vi "GetAction.vi"(0 "Check Condition":T16, 5 "Query Array":T17[](array[typedef]), 7 "input cluster":T1, 11 "error in (no error)":errorcluster) -> (3 "Compound AND":bool, 4 "Results Array":bool[](array[boolean]), 6 "Status Array Out":string[](array[string]), 13 "Convectron ATM Result Array":i32[](array[numeric]), 14 "Generate Event?":bool, 15 "error out":errorcluster)   [LabVIEW 2011]
uses:
  action_typdef.ctl
  Error codes.ctl
  MainCluster_typdef.ctl
  EC Status Named_typdef.ctl
  EC Statusboolarray2_typdef.ctl
  EC Statusboolarray3_typdef.ctl
  EC Statusboolarray1_typdef.ctl
  EC statusintegerarray_typdef.ctl
  EC statusfloatrarray_typdef.ctl
  LB Status Named_typdef.ctl
  LB Statusboolarray1_typdef.ctl
  LB Statusboolarray2_typdef.ctl
  LB Statusboolarray3_typdef.ctl
  LB statusintegerarray_typdef.ctl
  LB statusfloatrarray_typdef.ctl
  Chamber Selection_typdef.ctl
  GPM Mode_typdef.ctl
panel:
  out "Msg out":string
types:
  T1 = typedef "MainCluster_typdef.ctl" = cluster{"Isolate HPBD":bool, "Core":cluster{"Current VI Reference":refnum<vi>, "Close Panel on Exit?":bool}, "Status Display Array":string[], "Connection URLs":cluster{"Source_URL EC":string, "Target_URL EC":string, "Source_URL LB":string, "Target_URL LB":string}, "EC Status":cluster{"bits 2":bool[], "bits 2":bool[], "bits 2":bool[], i32[], "FLOAT NUMBERS 2":sgl[]}, "EC Status Named":T2, "TCPConnection":cluster{"Status TCP Connection EC":refnum<k5>, "Command TCP Connection EC":refnum<k5>, "Status TCP Connection LB":refnum<k5>, "Command TCP Connection LB":refnum<k5>}, "EC Command Cluster":cluster{"boolarray1":cluster{bool, bool, bool, bool, bool, bool, bool, bool, bool, bool, bool, bool, bool, bool, bool, bool}, "boolarray2":cluster{bool, bool, bool, bool, bool, bool, bool, bool, bool, bool, bool, bool, bool, bool, bool, bool}, "boolarray3":cluster{bool, bool, bool, bool, bool, bool, bool, bool, bool, bool, bool, bool, bool, bool, bool, bool}, "boolarray4":cluster{bool, bool, bool, bool, bool, bool, bool, bool, bool, bool, bool, bool, bool, bool, bool, bool}}, "EC Command Named":cluster{"EC Command array 1":cluster{"ROUGHING MANIFOLD VALVE":bool, "BACKING MANIFOLD VALVE":bool, "ROUGHING BACKING CONNECT VALVE":bool, "BTL ROUGHING VALVE":bool, "BTL VENT VALVE":bool, "BTL Turbo Gate Valve":bool, "BTL Turbo Backing Valve":bool, "Roughing Manifold VV":bool, "Backing Manifold VV":bool, "TARGET ROUGHING VALVE":bool, "BTL2 ROUGHING VALVE":bool, "HPD ROUGHING VALVE":bool, "GV BTL-TARGET":bool, "GV TARGET-BTL2":bool, "GV BTL2-HPD":bool, "TARGET VENT VALVE":bool}, " EC Command array 2":cluster{"BTL2 VENT VALVE":bool, "HPD VENT VALVE":bool, "TARGET  Turbo Gate Valve 1":bool, "TARGET  Turbo Gate Valve 2":bool, "BTL2 Turbo Gate Valve":bool, "HPD  Turbo Gate Valve":bool, "TARGET Turbo Backing Valve 1":bool, "TARGET Turbo Backing Valve 2":bool, "BTL2 Turbo Backing Valve":bool, "HPD Turbo Backing Valve":bool, "Spare 1":bool, "Spare 2":bool, "ROUGHING PUMP":bool, "BACKING PUMP":bool, "Spare 3":bool, "Spare 4":bool}, "EC Command array 3":cluster{"Spare 1":bool, "Spare 2":bool, "Spare 3":bool, "BTL Turbo Vent Valve":bool, "TARGET1 Turbo Vent Valve":bool, "TARGET2 Turbo Vent Valve":bool, "BTL2 Turbo Vent Valve":bool, "HPD Turbo Vent Valve":bool, "Spare 4":bool, "Spare 5":bool, "GPM":bool, "GVM":bool, "Spare 6":bool, "BTL turbo pump":bool, "TARGET1 turbo pump":bool, "TARGET2 turbo pump":bool}, "EC Command array 4":cluster{"BLT turbo pump":bool, "HPD turbo pump":bool, "Spare 1":bool, "BTL ION GAUGE ion gauge":bool, "BTL ION GAUGE  ion gauge degas":bool, "TARGET ion gauge":bool, "TARGET ion gauge degas":bool, "BTL2 ion gauge":bool, "BTL2 ion gauge degas":bool, "HPD ion gauge":bool, "HPD ion gauge degas":bool, "Spare 2":bool, "Spare 3":bool, "Spare 4":bool, "Spare 5":bool, "Spare 6":bool}}, "LB Status Named":T8, "LB Status":cluster{"bits 2":bool[], "bits 2":bool[], "bits 2":bool[], i32[], "FLOAT NUMBERS 2":sgl[]}, "LB Command Cluster":cluster{"boolarray1":cluster{bool, bool, bool, bool, bool, bool, bool, bool, bool, bool, bool, bool, bool, bool, bool, bool}, "boolarray2":cluster{bool, bool, bool, bool, bool, bool, bool, bool, bool, bool, bool, bool, bool, bool, bool, bool}, "boolarray3":cluster{bool, bool, bool, bool, bool, bool, bool, bool, bool, bool, bool, bool, bool, bool, bool, bool}, "boolarray4":cluster{bool, bool, bool, bool, bool, bool, bool, bool, bool, bool, bool, bool, bool, bool, bool, bool}}, "LB Command Named":cluster{"LB commandarray1":cluster{"ROUGHING MANIFOLD VALVE":bool, "BACKING MANIFOLD VALVE":bool, "ROUGHING BACKING CONNECT VALVE":bool, "COMPRESSOR ROUGHING VALVE":bool, "M123 ROUGHING VALVE":bool, "BEAMDUMP ROUGHING VALVE":bool, "OAP ROUGHING VALVE":bool, "GATE VALVE COMP-M123":bool, "GATE VALVE BEAM DUMP":bool, "GATE VALVE M123-OAP":bool, "GATE VALVE OAP-BTL":bool, "COMPRESSOR VENT VALVE":bool, "M123 VENT VALVE":bool, "BEAMDUMP VENT VALVE":bool, "OAP VENT VALVE":bool, "COMPRESSOR Turbo Gate Valve":bool}, "LB commandarray2":cluster{"M123 Turbo Gate Valve":bool, "OAP Turbo Gate Valve":bool, "COMPRESSOR Turbo Backing Valve":bool, "M123 Turbo Backing Valve":bool, "OAP Turbo Backing Valve":bool, "Roughing Manifold Vent Valve":bool, "Backing Manifold Vent Valve":bool, "Spare 1":bool, "Spare 2":bool, "Spare 3":bool, "Spare 4":bool, "Spare 5":bool, "ROUGHING PUMP":bool, "BACKING PUMP":bool, "Spare 6":bool, "Spare 7":bool}, "LB commandarray3":cluster{"Spare 1":bool, "Spare 2":bool, "Spare 3":bool, "COMP Turbo Vent Valve":bool, "M123 Turbo Vent Valve":bool, "OAP Turbo Vent Valve":bool, "Spare 4":bool, "Spare 5":bool, "Spare 6":bool, "Spare 7":bool, "GPM":bool, "GVM":bool, "Spare 8":bool, "COMP turbo pump":bool, "M123 turbo pump":bool, "OAP turbo pump":bool}, "LB commandarray4":cluster{"Spare 1":bool, "Spare 2":bool, "Spare 3":bool, "COMP ION GAUGE":bool, "COMP ION GAUGE degas":bool, "M123 ION GAUGE":bool, "M123 ION GAUGE degas":bool, "OAP ION GAUGE":bool, "OAP ION GAUGE degas":bool, "Spare 4":bool, "Spare 5":bool, "Spare 6":bool, "Spare 7":bool, "Spare 8":bool, "Spare 9":bool, "Spare 10":bool}}, "VI Refnum":refnum<vi>, "Chamber Selection":T14, "GPM Mode":T15, "Debug Mode?":bool, "State Sanity Check Array":bool[], "Critical Failures":cluster{"GPM Exit?":bool}, "Comm Ready?":bool, "Status Reconnect Attempt":dbl}
  T2 = typedef "EC Status Named_typdef.ctl" = cluster{"EC statusboolarray2":T3, "EC statusboolarray3":T4, "EC statusboolarray1":T5, "EC statusintegerarray":T6, "EC statusfloatarray":T7}
  T3 = typedef "EC Statusboolarray2_typdef.ctl" = cluster{"Spare 1":bool, "Spare 2":bool, "Spare 3":bool, "Spare 4":bool, "ROUGHING PUMP run opened":bool, "ROUGHING PUMP no fault closed":bool, "BACKING PUMP run opened":bool, "BACKING PUMP no fault closed":bool, "BTL TURBO turbo fault feedback":bool, "BTL TURBO turbo normal feedback":bool, "TARGET 1 TURBO turbo fault feedback":bool, "TARGET 1 TURBO turbo normal feedback":bool, "TARGET 2 TURBO turbo fault feedback":bool, "TARGET 2 TURBO turbo normal feedback":bool, "BTL2 TURBO turbo fault feedback":bool, "BTL2 TURBO turbo normal feedback":bool, "HPD TURBO turbo fault feedback":bool, "HPD TURBO turbo normal feedback":bool, "Spare 5":bool, "Spare 6":bool, "ROUGHING PUMP FLOW SWITCH":bool, "BACKING PUMP FLOW SWITCH":bool, "BTL TURBO FLOW SWITCH":bool, "TARGET 1 TURBO FLOW SWITCH":bool, "TARGET 2 TURBO FLOW SWITCH":bool, "BTL2 TURBO FLOW SWITCH":bool, "HPD TURBO FLOW SWITCH":bool, "Spare 7":bool, "BTL ion gauge on signal":bool, "BTL ion gauge degas signal":bool, "TARGET ion gauge on signal":bool, "TARGET ion gauge degas signal":bool, "BTL2 ion gauge on signal":bool, "BTL2 ion gauge degas signal":bool, "HPD ion gauge on signal":bool, "HPD ion gauge degas signal":bool, "Spare 8":bool, "Spare 9":bool, "Spare 10":bool, "Spare 11":bool, "ROUGHING MANIFOLD VALVE":bool, "BACKING MANIFOLD VALVE":bool, "ROUGHING BACKING CONNECT VALVE":bool, "BTL ROUGHING VALVE":bool, "BTL VENT VALVE":bool, "BTL Turbo Gate Valve":bool, "BTL Turbo Backing Valve":bool, "Roughing Manifold VV":bool, "Backing Manifold VV":bool, "TARGET ROUGHING VALVE":bool, "BTL2 ROUGHING VALVE":bool, "HPD ROUGHING VALVE":bool, "GV BTL-TARGET":bool, "GV TARGET-BTL2":bool, "GV BTL2-HPD":bool, "TARGET VENT VALVE":bool, "BTL2 VENT VALVE":bool, "HPD VENT VALVE":bool, "TARGET  Turbo Gate Valve 1":bool, "TARGET  Turbo Gate Valve 2":bool, "BTL2 Turbo Gate Valve":bool, "HPD  Turbo Gate Valve":bool, "TARGET Turbo Backing Valve 1":bool, "TARGET Turbo Backing Valve 2":bool}
  T4 = typedef "EC Statusboolarray3_typdef.ctl" = cluster{"BTL2 Turbo Backing Valve":bool, "HPD Turbo Backing Valve":bool, "Spare 1":bool, "Spare 2":bool, "Spare 3":bool, "Spare 4":bool, "Spare 5":bool, "Spare 6":bool, "Spare 7":bool, "Spare 8":bool, "Spare 9":bool, "BTL Turbo Vent Valve":bool, "TARGET1 Turbo Vent Valve":bool, "TARGET2 Turbo Vent Valve":bool, "BTL2 Turbo Vent Valve":bool, "HPD Turbo Vent Valve":bool, "Spare 10":bool, "Spare 11":bool, "BTL turbo pump run signal":bool, "TARGET1 turbo pump run signal":bool, "TARGET2 turbo pump run signal":bool, "BTL2 turbo pump run signal":bool, "HPD turbo pump run signal":bool, "Spare 12":bool, "watch dog timer - out":bool, "BTL vented – out":bool, "BTL medvac – out":bool, "BTL hivac – out":bool, "GPM EC - out":bool, "GVM EC - out":bool, "RP EC status - out":bool, "RP LB toggle - out":bool, "GATE ALL - closed out":bool, "Spare 13":bool, "Spare 14":bool, "Spare 15":bool, "Spare 16":bool, "Spare 17":bool, "Spare 18":bool, "Spare 19":bool, "Spare 20":bool, "Spare 21":bool, "Spare 22":bool, "Spare 23":bool, "Spare 24":bool, "Spare 25":bool, "Spare 26":bool, "Spare 27":bool}
  T5 = typedef "EC Statusboolarray1_typdef.ctl" = cluster{"BTL ion gauge on feedback":bool, "BTL ion gauge degas feedback":bool, "TARGET ion gauge on feedback":bool, "TARGET ion gauge degas feedback":bool, "BTL2 ion gauge on feedback":bool, "BTL2 ion gauge degas feedback":bool, "HPD ion gauge on feedback":bool, "HPD ion gauge degas feedback":bool, "Spare 1":bool, "Spare 2":bool, "Spare 3":bool, "Spare 4":bool, "ROUGHING MANIFOLD VALVE opened":bool, "ROUGHING MANIFOLD VALVE closed":bool, "BACKING MANIFOLD VALVE opened":bool, "BACKING MANIFOLD VALVE closed":bool, "ROUGHING BACKING CONNECT VALVE opened":bool, "ROUGHING BACKING CONNECT VALVE closed":bool, "BTL ROUGHING VALVE opened":bool, "BTL ROUGHING VALVE closed":bool, "BTL VENT VALVE opened":bool, "BTL VENT VALVE closed":bool, "BTL Turbo Gate Valve opened":bool, "BTL Turbo Gate Valve closed":bool, "BTL Turbo Backing Valve opened":bool, "BTL Turbo Backing Valve closed":bool, "Roughing Manifold VV opened":bool, "Roughing Manifold VV closed":bool, "Backing Manifold VV opened":bool, "Backing Manifold VV closed":bool, "TARGET ROUGHING VALVE opened":bool, "TARGET ROUGHING VALVE closed":bool, "BTL2 ROUGHING VALVE opened":bool, "BTL2 ROUGHING VALVE closed":bool, "HPD ROUGHING VALVE opened":bool, "HPD ROUGHING VALVE closed":bool, "GV BTL-TARGET opened":bool, "GV BTL-TARGET closed":bool, "GV TARGET-BTL2 opened":bool, "GV TARGET-BTL2 closed":bool, "GV BTL2-HPD opened":bool, "GV BTL2-HPD closed":bool, "TARGET VENT VALVE opened":bool, "TARGET VENT VALVE closed":bool, "BTL2 VENT VALVE opened":bool, "BTL2 VENT VALVE closed":bool, "HPD VENT VALVE opened":bool, "HPD VENT VALVE closed":bool, "TARGET  Turbo Gate Valve 1 opened":bool, "TARGET  Turbo Gate Valve 1 closed":bool, "TARGET  Turbo Gate Valve 2 opened":bool, "TARGET  Turbo Gate Valve 2 closed":bool, "BTL2 Turbo Gate Valve opened":bool, "BTL2 Turbo Gate Valve closed":bool, "HPD  Turbo Gate Valve opened":bool, "HPD  Turbo Gate Valve closed":bool, "TARGET Turbo Backing Valve 1 opened":bool, "TARGET Turbo Backing Valve 1 closed":bool, "TARGET Turbo Backing Valve 2 opened":bool, "TARGET Turbo Backing Valve 2 closed":bool, "BTL2 Turbo Backing Valve opened":bool, "BTL2 Turbo Backing Valve closed":bool, "HPD Turbo Backing Valve opened":bool, "HPD Turbo Backing Valve closed":bool}
  T6 = typedef "EC statusintegerarray_typdef.ctl" = cluster{"BTL vacuum status word convectron ATM":i32, "TARGET vacuum status word convectron ATM 2":i32, "BTL2 vacuum status word convectron ATM 3":i32, "HPD vacuum status word convectron ATM 4":i32, "Spare 1":i32, "Spare 2":i32, "roughing pump vacuum status word convectron":i32, "backing pump vacuum status word convectron":i32, "roughing manifold vacuum status word convectron":i32, "backing manifold vacuum status word convectron":i32, "BTL Convectron vacuum status word convectron":i32, "TARGET1 Convectron vacuum status word convectron":i32, "TARGET2 Convectron vacuum status word convectron":i32, "BTL2 Convectron vacuum status word convectron":i32, "HPD Convectron vacuum status word convectron":i32, "BTL status word turbo pump":i32, "TARGET1 status word turbo pump":i32, "TARGET2 status word turbo pump":i32, "BTL2 status word turbo pump??":i32, "HPD status word turbo pump":i32, "Spare 3":i32, "Spare 4":i32, "Spare 5":i32, "Spare 6":i32, "BTL CONVECTRON Consolidate":i32, "Spare 7":i32, "Spare 8":i32, "Spare 9":i32, "TARGET Consolidate":i32, "Spare 10":i32, "Spare 11":i32, "Spare 12":i32, "BTL2 Consolidate":i32, "Spare 13":i32, "Spare 14":i32, "Spare 15":i32, "HPD Consolidate":i32, "Spare 16":i32, "Spare 17":i32, "Spare 18":i32, "Spare 19":i32, "Spare 20":i32, "Spare 21":i32, "Spare 22":i32, "Spare 23":i32, "Spare 24":i32, "Spare 25":i32, "Spare 26":i32}
  T7 = typedef "EC statusfloatrarray_typdef.ctl" = cluster{"BTL READING ION GAUGE":dbl, "TARGET READING ION GAUGE":dbl, "BTL2 READING ION GAUGE":dbl, "HPD READING ION GAUGE":dbl, "Spare 1":dbl, "Spare 2":dbl, "Spare 3":dbl, "Spare 4":dbl, "roughing pump READING CONVECTRON GAUGE":dbl, "backing pump READING CONVECTRON GAUGE":dbl, "roughing manifold READING CONVECTRON GAUGE":dbl, "backing manifold READING CONVECTRON GAUGE":dbl, "BTL Convectron READING CONVECTRON GAUGE":dbl, "TARGET1 READING CONVECTRON GAUGE":dbl, "TARGET2 READING CONVECTRON GAUGE":dbl, "BTL2 READING CONVECTRON GAUGE":dbl, "HPD READING CONVECTRON GAUGE":dbl, "Spare 5":dbl, "Spare 6":dbl, "Spare 7":dbl, "Spare 8":dbl, "Spare 9":dbl, "Spare 10":dbl, "Spare 11":dbl}
  T8 = typedef "LB Status Named_typdef.ctl" = cluster{"LB statusboolarray1":T9, "LB statusboolarray2":T10, "LB statusboolarray3":T11, "LB statusintegerarray":T12, "LB statusfloatarray":T13}
  T9 = typedef "LB Statusboolarray1_typdef.ctl" = cluster{"COMP ion gauge on feedback":bool, "COMP ion gauge degas feedback":bool, "M123 ion gauge on feedback":bool, "M123 ion gauge degas feedback":bool, "OAP ion gauge on feedback":bool, "OAP ion gauge degas feedback":bool, "Spare 1":bool, "Spare 2":bool, "Spare 3":bool, "Spare 4":bool, "Spare 5":bool, "Spare 6":bool, "ROUGHING MANIFOLD VALVE opened":bool, "ROUGHING MANIFOLD VALVE closed":bool, "BACKING MANIFOLD VALVE opened":bool, "BACKING MANIFOLD VALVE closed":bool, "ROUGHING BACKING CONNECT VALVE opened":bool, "ROUGHING BACKING CONNECT VALVE closed":bool, "COMPRESSOR ROUGHING VALVE opened":bool, "COMPRESSOR ROUGHING VALVE closed":bool, "M123 ROUGHING VALVE opened":bool, "M123 ROUGHING VALVE closed":bool, "BEAMDUMP ROUGHING VALVE opened":bool, "BEAMDUMP ROUGHING VALVE closed":bool, "OAP ROUGHING VALVE opened":bool, "OAP ROUGHING VALVE closed":bool, "GATE VALVE COMP-M123 opened":bool, "GATE VALVE COMP-M123 closed":bool, "GATE VALVE BEAM DUMP opened":bool, "GATE VALVE BEAM DUMP closed":bool, "GATE VALVE M123-OAP opened":bool, "GATE VALVE M123-OAP closed":bool, "GATE VALVE OAP-BTL opened":bool, "GATE VALVE OAP-BTL closed":bool, "COMPRESSOR VENT VALVE opened":bool, "COMPRESSOR VENT VALVE closed":bool, "M123 VENT VALVE opened":bool, "M123 VENT VALVE closed":bool, "BEAMDUMP VENT VALVE opened":bool, "BEAMDUMP VENT VALVE closed":bool, "OAP VENT VALVE opened":bool, "OAP VENT VALVE closed":bool, "COMPRESSOR Turbo Gate Valve opened ":bool, "COMPRESSOR Turbo Gate Valve closed":bool, "M123 Turbo Gate Valve opened":bool, "M123 Turbo Gate Valve closed":bool, "OAP Turbo Gate Valve opened":bool, "OAP Turbo Gate Valve closed":bool, "COMPRESSOR Turbo Backing Valve opened":bool, "COMPRESSOR Turbo Backing Valve closed":bool, "M123 Turbo Backing Valve opened":bool, "M123 Turbo Backing Valve closed":bool, "OAP Turbo Backing Valve opened":bool, "OAP Turbo Backing Valve closed":bool, "Roughing Manifold Vent Valve opened":bool, "Roughing Manifold Vent Valve closed":bool, "Spare 7":bool, "Spare 8":bool, "Spare 9":bool, "Spare 10":bool, "RP RUN opened":bool, "RP no FAULT closed":bool, "BP RUN opened":bool, "BP no FAULT closed":bool}
  T10 = typedef "LB Statusboolarray2_typdef.ctl" = cluster{"Spare 1":bool, "Spare 2":bool, "Spare 3":bool, "Spare 4":bool, "ROUGHING PUMP run":bool, "ROUGHING PUMP no fault":bool, "BACKING PUMP run":bool, "BACKING PUMP no fault":bool, "COMP TURBO fault feedback":bool, "COMP TURBO normal feedback":bool, "M123 TURBO fault feedback":bool, "M123 TURBO normal feedback":bool, "OAP TURBO fault feedback":bool, "OAP TURBO normal feedback":bool, "Spare 9":bool, "Spare 10":bool, "Spare 11":bool, "Spare 12":bool, "Spare 13":bool, "Spare 14":bool, "ROUGHING PUMP FLOW SWITCH":bool, "BACKING PUMP FLOW SWITCH":bool, "COMP TURBO FLOW SWITCH":bool, "M123 TURBO FLOW SWITCH":bool, "OAP TURBO FLOW SWITCH":bool, "Spare 15":bool, "Spare 16":bool, "Spare 17":bool, "COMP ion gauge on signal":bool, "COMP ion gauge degas signal":bool, "M123 ion gauge on signal":bool, "M123 ion gauge degas signal":bool, "OAP ion gauge on signal":bool, "OAP ion gauge degas signal":bool, "Spare 18":bool, "Spare 19":bool, "Spare 20":bool, "Spare 21":bool, "Spare 22":bool, "Spare 23":bool, "ROUGHING MANIFOLD VALVE":bool, "BACKING MANIFOLD VALVE":bool, "ROUGHING BACKING CONNECT VALVE":bool, "COMPRESSOR ROUGHING VALVE":bool, "M123 ROUGHING VALVE":bool, "BEAMDUMP ROUGHING VALVE":bool, "OAP ROUGHING VALVE":bool, "GATE VALVE COMP-M123":bool, "GATE VALVE BEAM DUMP":bool, "GATE VALVE M123-OAP":bool, "GATE VALVE OAP-BTL":bool, "COMPRESSOR VENT VALVE":bool, "M123 VENT VALVE":bool, "BEAMDUMP VENT VALVE":bool, "OAP VENT VALVE":bool, "COMPRESSOR Turbo Gate Valve":bool, "M123 Turbo Gate Valve":bool, "OAP Turbo Gate Valve":bool, "COMPRESSOR Turbo Backing Valve":bool, "M123 Turbo Backing Valve":bool, "OAP Turbo Backing Valve":bool, "Spare 24":bool, "Spare 25":bool, "Spare 26":bool}
  T11 = typedef "LB Statusboolarray3_typdef.ctl" = cluster{"Spare 1":bool, "Spare 2":bool, "Spare 3":bool, "Spare 4":bool, "ROUGHING PUMP":bool, "BACKING PUMP":bool, "Spare 5":bool, "Spare 6":bool, "Spare 7":bool, "Spare 8":bool, "Spare 9":bool, "COMP Turbo Vent Valve":bool, "M123 Turbo Vent Valve":bool, "OAP Turbo Vent Valve":bool, "Spare 10":bool, "Spare 11":bool, "Spare 12":bool, "Spare 13":bool, "COMP turbo pump run signal":bool, "M123 turbo pump run signal":bool, "OAP turbo pump run signal":bool, "Spare 14":bool, "Spare 15":bool, "Spare 16":bool, "watch dog timer - out":bool, "GATE OAP-BTL - closed out":bool, "GATE 1 – closed out":bool, "GATE 2 – closed out":bool, "GATE 3,4 – closed out":bool, "GPM LB - out":bool, "GVM LB - out":bool, "RP LB status - out":bool, "RP EC - toggle - out":bool, "Spare 17":bool, "Spare 18":bool, "Spare 19":bool, "Spare 20":bool, "Spare 21":bool, "Spare 22":bool, "Spare 23":bool}
  T12 = typedef "LB statusintegerarray_typdef.ctl" = cluster{"COMP vacuum status word convectron ATM":i32, "M123 vacuum status word convectron ATM":i32, "OAP vacuum status word convectron ATM":i32, "HPBD vacuum status word convectron ATM":i32, "Spare 1":i32, "Spare 2":i32, "roughing pump vacuum status word convectron":i32, "backing pump vacuum status word convectron":i32, "roughing manifold vacuum status word convectron":i32, "backing manifold vacuum status word convectron":i32, "COMP Convectron vacuum status word convectron":i32, "M123 Convectron vacuum status word convectron":i32, "OAP Convectron vacuum status word convectron":i32, "Spare 3":i32, "Spare 4":i32, "COMP status word turbo pump":i32, "M123 status word turbo pump":i32, "OAP status word turbo pump":i32, "Spare 5":i32, "Spare 6":i32, "Spare 7":i32, "Spare 8":i32, "Spare 9":i32, "Spare 10":i32, "COMP CONVECTRON consloidate":i32, "Spare 11":i32, "Spare 12":i32, "Spare 13":i32, "M123 CONVECTRON consloidate":i32, "Spare 14":i32, "Spare 15":i32, "Spare 16":i32, "OAP CONVECTRON consloidate":i32, "Spare 17":i32, "Spare 18":i32, "Spare 19":i32, "HPBD CONVECTRON consloidate":i32, "Spare 20":i32, "Spare 21":i32, "Spare 22":i32, "Spare 23":i32, "Spare 24":i32, "Spare 25":i32, "Spare 26":i32, "Spare 27":i32, "Spare 28":i32, "Spare 29":i32, "Spare 30":i32}
  T13 = typedef "LB statusfloatrarray_typdef.ctl" = cluster{"COMP READING ION GAUGE":dbl, "M123 READING ION GAUGE":dbl, "OAP READING ION GAUGE":dbl, "Spare 1":i32, "Spare 2":i32, "Spare 3":i32, "Spare 4":i32, "Spare 5":i32, "roughing pump CONVECTRON GAUGE":dbl, "backing pump CONVECTRON GAUGE":dbl, "roughing manifold CONVECTRON GAUGE":dbl, "backing manifold CONVECTRON GAUGE":dbl, "COMP Convectron CONVECTRON GAUGE":dbl, "M123 Convectron CONVECTRON GAUGE":dbl, "OAP Convectron CONVECTRON GAUGE":dbl, "Spare 6":i32, "Spare 7":i32, "Spare 8":i32, "Spare 9":i32, "Spare 10":i32, "Spare 11":i32, "Spare 12":i32, "Spare 13":i32, "Spare 14":i32}
  T14 = typedef "Chamber Selection_typdef.ctl" = cluster{"COMP":bool, "M123":bool, "HPBD":bool, "OAP":bool, "BTL":bool, "TARGET":bool, "BTL2":bool, "HPD":bool}
  T15 = typedef "GPM Mode_typdef.ctl" = enum16{"Complete Global Pump Mode", "Selected Global Pump Mode"}
  T16 = typedef "Error codes.ctl" = enum16{"001-GPM and GVM conditions", "002-Turbo gate valve status", "003-Chamber Gate Valve Status", "004-Check Chamber Pressures", "005-Check GPM Handshake", "006-Roughing Pump Status", "007-Backing Pump Status", "008-Backing valve status", "009-Roughing Manifold Pressure Status", "010-Roughing Valve Status", "011-Roughing Pump Status", "012-Turbo Backing Valve Status", "013-MID-VAC Status", "999-No Event"}
  T17 = typedef "action_typdef.ctl" = enum16{"No Action", "Is EC GPM Mode ON?", "Is EC GPM Mode Off?", "Is EC GVM Mode ON?", "Is EC GVM Off?", "Is  EC GPM or GVM Mode ON?", "Is LB GPM Mode ON?", "Is LB GPM Mode Off?", "Is LB GVM Mode ON?", "Is LB GVM Mode Off?", "Is  LB GPM or GVM Mode ON?", "Is M123 Turbo Gate Valve Opened? ", "Is M123 Turbo Gate Valve Closed?", "Is OAP Turbo Gate Valve Opened?", "Is OAP Turbo Gate Valve Closed?", "Is BTLTurbo Gate Valve Opened?", "Is BTL Turbo Gate Valve Closed?", "Is TARGET Turbo Gate Valve 1Opened?", "Is TARGET1 Turbo Gate Valve Closed?", "Is TARGET Turbo Gate Valve 2 Opened?", "Is TAREGT2 Turbo Gate Valve Closed?", "Is BTL2 Turbo Gate Valve Opened?", "Is BTL2 Turbo Gate Valve Closed?", "Is HPD Turbo Gate Valve Opened?", "Is HPD Turbo Gate Valve Closed?", "Is COMP to M123 gate Valve Opened?", "Is COMP to M123 Valve Closed?", "Is HPBD Gate Valve Opened?", "Is HPBD Gate Valve Closed?", "Is M123 to OAP gate valve opened?", "Is M123 to OAP gate valve closed?", "Is OAP to BLT gate valve opened?", "Is OAP to BTL Gate Valve Closed?", "Is BLT to TARGET gate valve opened?", "Is BTL to TARGET Gate Valve Closed?", "Is TARGET to BLT2 gate valve opened?", "Is TARGET to BTL2 Gate Valve Closed?", "Is BLT2 to HPD gate valve opened?", "Is BTL2 to HPD Gate Valve Closed?", "Is COMP at Atmospheric Pressure?", "Is M123 at Atmospheric Pressure?", "Is BeamDump at Atmospheric Pressure?", "Is OAP at Atmospheric Pressure?", "Is BLT at Atmospheric Pressure", "Is TARGET at Atmospheric Pressure?", "Is BLT2 at Atmospheric Pressure?", "Is HPD at Atmospheric Pressure?", "Is the EC Roughing Pump ON?", "Is the EC Roughing Pump OFF?", "Does the EC Roughing Pump have a fault?", "Is the LB Roughing Pump ON?", "Is the LB Roughing Pump Off?", "Does the LB Roughing Pump have a fault?", "Is the EC Backing Pump ON?", "Is the EC Backing Pump OFF?", "Is the LB Backing Pump ON?", "Is the LB Backing Pump OFF?", "Does the EC Backing Pump have a fault?", "Does the LB Backing Pump have a fault?", "Is the EC Backing Pipe at Atmospheric Pressure", "Is the LB Backing Pipe at Atmospheric Pressure", "Is the EC Backing Manifold at Atmospheric Pressure", "s the LB Backing Manifold at Atmospheric Pressure?", "Is the EC Roughing Pipe at Atmospheric Pressure", "Is the LB Roughing Pipe at Atmospheric Pressure?", "Is the EC Roughing Manifold at Atmospheric Pressure", "Is the LB Roughing Manifold at Atmospheric Pressure", "Is LB Backing Manifold Valve Opened?", "Is EC Backing Manifold Valve Opened?", "Is LB Roughing Manifold Valve Opened?", "Is EC Roughing Manifold Valve Opened?", "Is COMP Roughing Valve Opened?", "Is M123 Roughing Valve Opened?", "Is M123 Roughing Valve Closed?", "Is OAP Roughing Valve Opened?", "Is OAP Roughing Valve Closed?", "Is HPBD Roughing Valve Opened?", "Is HPBD Roughing Valve Closed?", "Is BTL Roughing Valve Opened?", "Is BTL Roughing Valve Closed?", "Is TARGET Roughing Valve Opened?", "Is TARGET Roughing Valve Closed?", "Is BTL2 Roughing Valve Opened?", "Is BTL2 Roughing Valve Closed?", "Is HPD Roughing Valve Opened?", "Is HPD Roughing Valve Closed?", "Is COMP Turbo Backing Valve Opened?", "Is M123 Turbo Backing Valve Opened", "Is HPBD Turbo Backing Valve Opened?", "Is OAP Turbo Backing Valve Opened?", "Is BTL Turbo Backing Valve Opened?", "Is TARGET1 Turbo Backing Valve Opened?", "Is TARGET2 Turbo Backing Valve Opened?", "Is BTL2 Turbo Backing Valve Opened?", "Is HPD Turbo Backing Valve Opened?", "Is M123 Backing at MID-VAC?", "Is OAP Backing at MID-VAC?", "Is TARGET1 Backing at MID-VAC?", "Is TARGET2 Backing at MID-VAC?", "Is BTL Backing at MID-VAC?", "Is BTL2 Backing at MID-VAC?", "Is HPD Backing at MID-VAC?", "Is M123 Turbo in Normal Operation", "Is COMP Turbo in Normal Operation", "Is OAP Turbo in Normal Operation", "Is BTL Turbo in Normal Operation", "Is TARGET1 Turbo in Normal Operation", "Is TARGET2 Turbo in Normal Operation", "Is BTL2 Turbo in Normal Operation", "Is HPD Turbo in Normal Operation", "Is M123 at MID-VAC?", "Is OAP at MID-VAC?", "Is COMP at MID-VAC?", "Is BTL at MID-VAC?", "Is TARGET at MID-VAC?", "Is BTL2 at MID-VAC?", "Is HPD at MID-VAC?"}
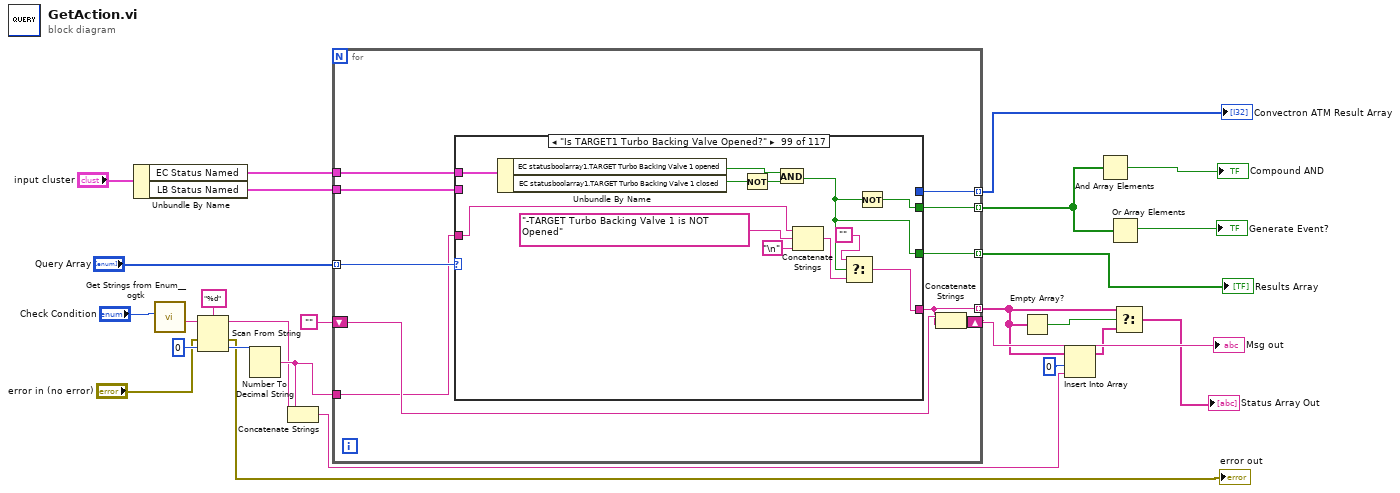
[diagram p0: block diagram]
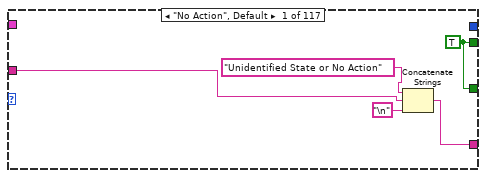
[diagram p2: hidden frame]
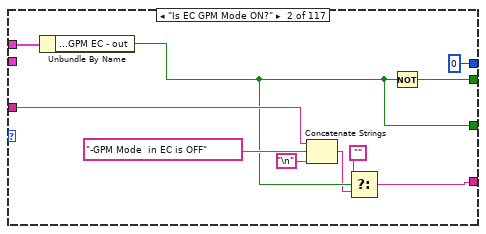
[diagram p3: hidden frame]
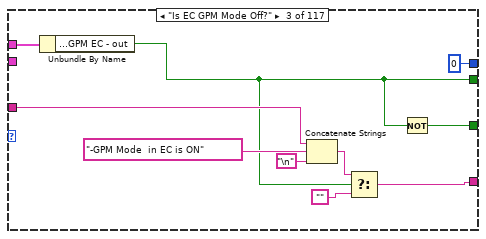
[diagram p4: hidden frame]
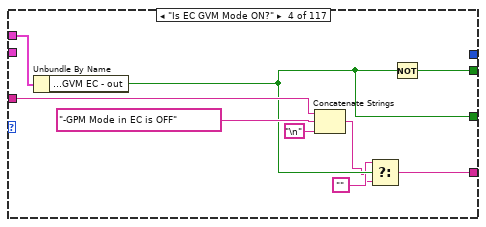
[diagram p5: hidden frame]
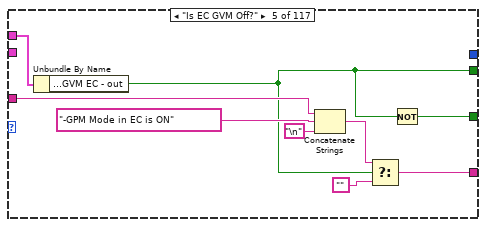
[diagram p6: hidden frame]
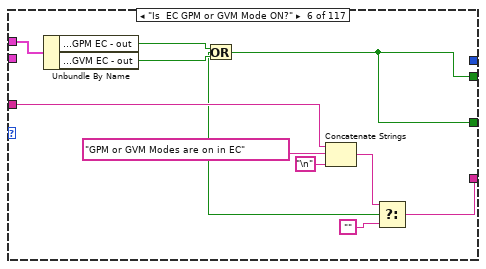
[diagram p7: hidden frame]
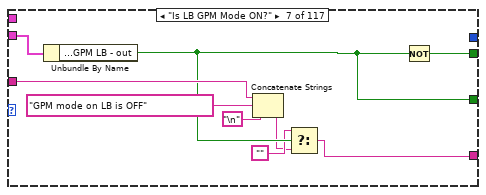
[diagram p8: hidden frame]
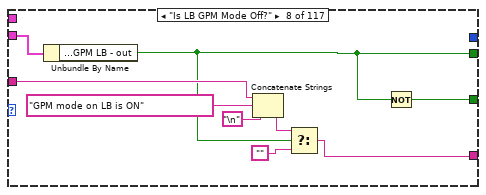
[diagram p9: hidden frame]
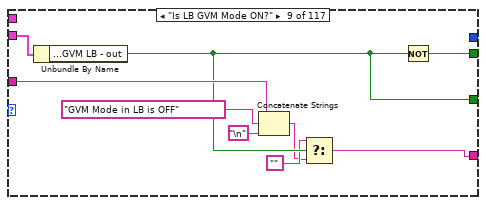
[diagram p10: hidden frame]
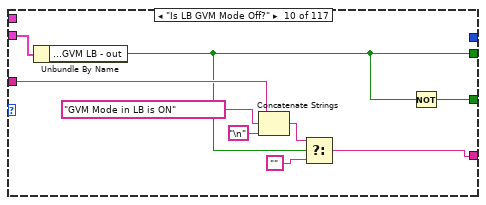
[diagram p11: hidden frame]
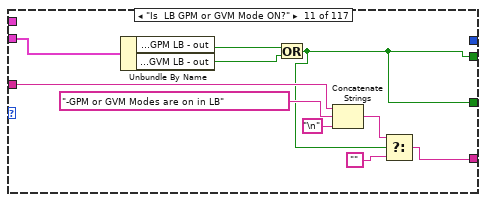
[diagram p12: hidden frame]
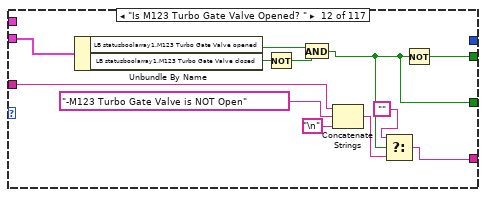
[diagram p13: hidden frame]
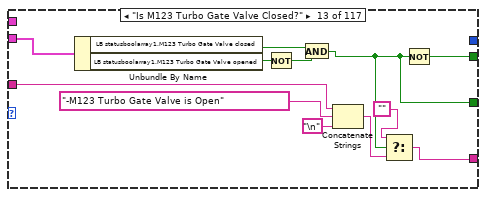
[diagram p14: hidden frame]
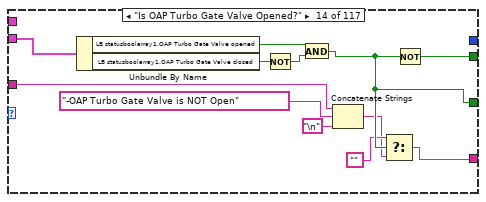
[diagram p15: hidden frame]
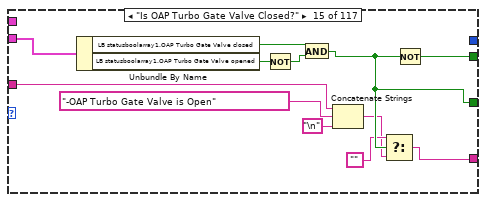
[diagram p16: hidden frame]
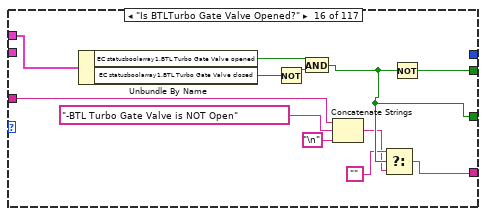
[diagram p17: hidden frame]
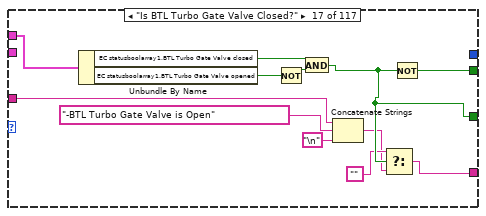
[diagram p18: hidden frame]
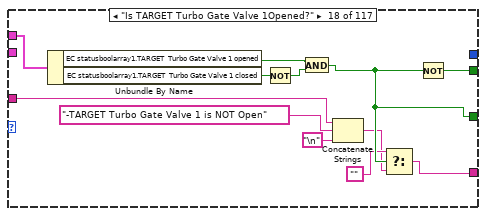
[diagram p19: hidden frame]
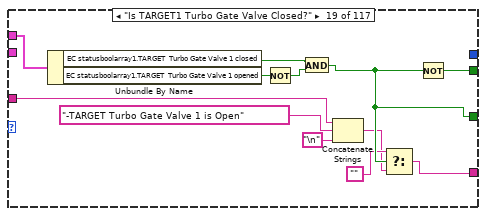
[diagram p20: hidden frame]
diagram:
  n1 = Unbundle By Name("input cluster") -> ("EC Status Named"=w26:T2, "LB Status Named"=w25:T8)
  n2 = call <userlib>:"Get Strings from Enum__ogtk.vi"("Enum"="Check Condition") -> ("String Value"=w20:string)  [unwired: 7 in, 3 out]
  n3 = Scan From String(format string="%d", input string=w20, error in="error in (no error)", default 1=0) -> (remaining string=w8:string, error out=→"error out":errorcluster, output 1=w17:i32)  [unwired: 1 in, 1 out]
  n4 = Number To Decimal String(number=w17) -> (decimal integer string=w9:string)  [unwired: 1 in]
  n5 = Concatenate Strings(w9, w8) -> (w7:string)
  n6 = for {
    tunnel: w26 -> [w36]
    tunnel: w25 -> [w35]
    tunnel: "Query Array" -> [w34] mode=indexing
    tunnel: [w33] -> w6 mode=indexing
    shift-right: [w30] -> w22
    shift-left: "" -> [w32]
    tunnel: [w31] -> w12 mode=indexing
    tunnel: w9 -> [w29]
    tunnel: [w28] -> w4 mode=indexing
    tunnel: [w27] -> w1 mode=indexing
    n7 = case shown="\"Is TARGET1 Turbo Backing Valve Opened?\"" w34 {
      tunnel: w36 -> [_ w51 w61 w70 w79 w89 _ _ _ _ _ _ _ _ _ w190 w202 w214 w226 w238 w250 w262 w274 w286 w298 _ _ _ _ _ _ _ _ w404 w416 w428 w440 w452 w464 _ _ _ _ _ _ _ w547 w559 w568 w580 w589 w601 w610 w622 w633 w642 w651 w660 _ _ _ _ w704 w712 _ _ w737 w747 _ _ w778 w788 _ w808 _ _ w841 w853 _ _ _ _ _ _ _ w947 w959 w971 w983 w995 w1007 w1019 w1031 _ _ _ _ w1092 w1104 w1116 w1128 w1140 _ _ w1172 w1183 w1194 w1205 w1216 _ _ _ w1260 w1271 w1282 w1293 w1304]
      tunnel: w35 -> [_ _ _ _ _ _ w98 w107 w116 w125 w135 w143 w155 w167 w179 _ _ _ _ _ _ _ _ _ _ w308 w320 w332 w344 w356 w368 w380 w392 _ _ _ _ _ _ w477 w488 w499 w509 w519 w529 w540 _ _ _ _ _ _ _ _ _ _ _ _ w669 w676 w687 w696 _ _ w718 w726 _ _ w755 w765 _ _ w795 _ w819 w831 _ _ w863 w875 w890 w899 w911 w923 w935 _ _ _ _ _ _ _ _ w1043 w1055 w1067 w1080 _ _ _ _ _ w1152 w1163 _ _ _ _ _ w1227 w1238 w1249 _ _ _ _ _]
      tunnel: [w41 w42 w53 w62 w72 w80 w90 w100 w108 w118 w126 w136 w148 w162 w174 w186 w198 w210 w222 w234 w246 w258 w270 w282 w294 w306 w318 w328 w340 w352 w364 w376 w388 w400 w412 w424 w436 w448 w460 w472 w482 w494 w506 w514 w524 w534 w545 w555 w566 w576 w587 w597 w608 w618 w630 w639 w650 w659 w668 w675 w685 w693 w701 w709 w717 w725 w733 w743 w753 w763 w773 w783 w793 w803 w813 w825 w837 w849 w861 w873 w885 w897 w909 w921 w933 w945 w957 w969 w981 w993 w1005 w1017 w1029 w1042 w1054 w1065 w1078 w1090 w1102 w1114 w1126 w1138 w1153 w1164 w1175 w1186 w1197 w1208 w1219 w1230 w1241 w1252 w1263 w1274 w1285 w1296 w1307] -> w33
      tunnel: [w37 w50 w59 w69 w77 w85 w97 w105 w115 w123 w131 w147 w159 w171 w183 w195 w207 w219 w231 w243 w255 w267 w279 w291 w303 w315 w327 w339 w351 w363 w375 w387 w399 w411 w423 w435 w447 w459 w471 w481 w492 w503 w513 w523 w533 w544 w554 w565 w575 w586 w596 w607 w617 w628 w637 w646 w655 w664 w673 w682 w691 w700 w708 w716 w724 w732 w735 w745 w756 w766 w775 w785 w796 w805 w817 w829 w842 w854 w866 w878 w893 w902 w914 w926 w938 w950 w962 w974 w986 w998 w1010 w1022 w1034 w1046 w1058 "" w1079 w1091 w1103 w1115 w1127 w1139 w1154 w1165 w1176 w1187 w1198 w1209 w1220 w1231 w1242 w1253 w1264 w1275 w1286 w1297 w1308] -> w31
      tunnel: w29 -> [w38 w47 w55 w66 w73 w81 w94 w101 w112 w119 w127 w144 w156 w168 w180 w192 w204 w216 w228 w240 w252 w264 w276 w288 w300 w312 w324 w336 w348 w360 w372 w384 w396 w408 w420 w432 w444 w456 w468 w478 w489 w500 w510 w520 w530 w541 w551 w562 w572 w583 w593 w604 w614 w625 w634 w643 w652 w661 w670 w679 w688 w697 w705 w713 w721 w729 w738 w748 w758 w768 w777 w787 w798 w807 w818 w830 w843 w855 w867 w879 w894 w903 w915 w927 w939 w951 w963 w975 w987 w999 w1011 w1023 w1035 w1047 w1059 w1071 w1083 w1095 w1107 w1119 w1131 w1143 w1157 w1168 w1179 w1190 w1201 w1212 w1223 w1234 w1245 w1256 w1267 w1278 w1289 w1300 w1311]
      tunnel: [_ 0 ("M123 vacuum status word convectron ATM") 0 ("M123 vacuum status word convectron ATM") _ _ _ _ _ _ _ _ _ _ _ _ _ _ _ _ _ _ _ _ _ _ _ _ _ _ _ _ _ _ _ _ _ _ _ _ w474 w485 w496 w508 w518 w528 w537 w550 w558 w571 w579 w592 w600 w613 w621 _ _ _ _ _ _ _ _ _ _ _ _ w736 w746 w757 w767 w776 w786 w797 w806 _ _ _ _ _ _ _ _ _ _ _ _ _ _ _ _ _ _ _ _ _ _ _ _ _ _ _ _ w1150 w1161 w1173 w1184 w1195 w1206 w1217 w1228 w1239 w1250 w1261 w1272 w1283 w1294 w1305] -> w28
      tunnel: [w41 w45 w52 w65 w71 w80 w93 w99 w111 w117 w126 w139 w151 w163 w175 w187 w199 w211 w223 w235 w247 w259 w271 w283 w295 w307 w319 w331 w343 w355 w367 w377 w389 w403 w415 w427 w439 w451 w463 w473 w483 w493 w507 w515 w525 w535 w546 w556 w567 w577 w588 w598 w609 w619 w629 w638 w647 w657 w665 w674 w686 w692 w701 w709 w717 w725 w734 w744 w754 w764 w774 w784 w794 w804 w814 w826 w838 w850 w862 w874 w889 w898 w910 w922 w934 w946 w958 w970 w982 w994 w1006 w1018 w1030 w1041 w1053 w1065 w1077 w1089 w1101 w1113 w1125 w1137 w1149 w1160 w1171 w1182 w1193 w1204 w1215 w1226 w1237 w1248 w1259 w1270 w1281 w1292 w1303] -> w27
      frame "No Action", Default {
        w41 = TRUE ("BACKING PUMP no fault")
        n8 = Concatenate Strings("Unidentified State or No Action", w38, "\n") -> (w37:string)
      }
      frame "Is EC GPM Mode ON?" {
        n9 = Unbundle By Name(w51) -> ("EC statusboolarray3.GPM EC - out"=w45:bool)
        n10 = Concatenate Strings(w47, "-GPM Mode  in EC is OFF", "\n") -> (w43:string)
        n11 = Select(t="", s=w45, f=w43) -> (s? t:f=w50:string)
        n12 = Not(x=w45) -> (.not. x?=w42:bool)
      }
      frame "Is EC GPM Mode Off?" {
        n13 = Unbundle By Name(w61) -> ("EC statusboolarray3.GPM EC - out"=w53:bool)
        n14 = Concatenate Strings(w55, "-GPM Mode  in EC is ON", "\n") -> (w56:string)
        n15 = Select(t=w56, s=w53, f="") -> (s? t:f=w59:string)
        n16 = Not(x=w53) -> (.not. x?=w52:bool)
      }
      frame "Is EC GVM Mode ON?" {
        n17 = Unbundle By Name(w70) -> ("EC statusboolarray3.GVM EC - out"=w65:bool)
        n18 = Concatenate Strings(w66, "-GPM Mode in EC is OFF", "\n") -> (w63:string)
        n19 = Select(t="", s=w65, f=w63) -> (s? t:f=w69:string)
        n20 = Not(x=w65) -> (.not. x?=w62:bool)
      }
      frame "Is EC GVM Off?" {
        n21 = Unbundle By Name(w79) -> ("EC statusboolarray3.GVM EC - out"=w72:bool)
        n22 = Concatenate Strings(w73, "-GPM Mode in EC is ON", "\n") -> (w74:string)
        n23 = Select(t=w74, s=w72, f="") -> (s? t:f=w77:string)
        n24 = Not(x=w72) -> (.not. x?=w71:bool)
      }
      frame "Is  EC GPM or GVM Mode ON?" {
        n25 = Unbundle By Name(w89) -> ("EC statusboolarray3.GPM EC - out"=w88:bool, "EC statusboolarray3.GVM EC - out"=w87:bool)
        n26 = Or(x=w88, y=w87) -> (x .or. y?=w80:bool)
        n27 = Concatenate Strings(w81, "GPM or GVM Modes are on in EC", "\n") -> (w82:string)
        n28 = Select(t=w82, s=w80, f="") -> (s? t:f=w85:string)
      }
      frame "Is LB GPM Mode ON?" {
        n29 = Unbundle By Name(w98) -> ("LB statusboolarray3.GPM LB - out"=w93:bool)
        n30 = Concatenate Strings(w94, "GPM mode on LB is OFF", "\n") -> (w91:string)
        n31 = Select(t="", s=w93, f=w91) -> (s? t:f=w97:string)
        n32 = Not(x=w93) -> (.not. x?=w90:bool)
      }
      frame "Is LB GPM Mode Off?" {
        n33 = Unbundle By Name(w107) -> ("LB statusboolarray3.GPM LB - out"=w100:bool)
        n34 = Concatenate Strings(w101, "GPM mode on LB is ON", "\n") -> (w102:string)
        n35 = Select(t=w102, s=w100, f="") -> (s? t:f=w105:string)
        n36 = Not(x=w100) -> (.not. x?=w99:bool)
      }
      frame "Is LB GVM Mode ON?" {
        n37 = Unbundle By Name(w116) -> ("LB statusboolarray3.GVM LB - out"=w111:bool)
        n38 = Concatenate Strings(w112, "GVM Mode in LB is OFF", "\n") -> (w109:string)
        n39 = Select(t="", s=w111, f=w109) -> (s? t:f=w115:string)
        n40 = Not(x=w111) -> (.not. x?=w108:bool)
      }
      frame "Is LB GVM Mode Off?" {
        n41 = Unbundle By Name(w125) -> ("LB statusboolarray3.GVM LB - out"=w118:bool)
        n42 = Concatenate Strings(w119, "GVM Mode in LB is ON", "\n") -> (w120:string)
        n43 = Select(t=w120, s=w118, f="") -> (s? t:f=w123:string)
        n44 = Not(x=w118) -> (.not. x?=w117:bool)
      }
      frame "Is  LB GPM or GVM Mode ON?" {
        n45 = Unbundle By Name(w135) -> ("LB statusboolarray3.GPM LB - out"=w133:bool, "LB statusboolarray3.GVM LB - out"=w134:bool)
        n46 = Or(x=w133, y=w134) -> (x .or. y?=w126:bool)
        n47 = Concatenate Strings(w127, "-GPM or GVM Modes are on in LB", "\n") -> (w128:string)
        n48 = Select(t=w128, s=w126, f="") -> (s? t:f=w131:string)
      }
      frame "Is M123 Turbo Gate Valve Opened? " {
        n49 = Unbundle By Name(w143) -> ("LB statusboolarray1.M123 Turbo Gate Valve opened"=w140:bool, "LB statusboolarray1.M123 Turbo Gate Valve closed"=w142:bool)
        n50 = Not(x=w142) -> (.not. x?=w141:bool)
        n51 = And(x=w140, y=w141) -> (x .and. y?=w139:bool)
        n52 = Concatenate Strings(w144, "-M123 Turbo Gate Valve is NOT Open", "\n") -> (w137:string)
        n53 = Select(t="", s=w139, f=w137) -> (s? t:f=w147:string)
        n54 = Not(x=w139) -> (.not. x?=w136:bool)
      }
      frame "Is M123 Turbo Gate Valve Closed?" {
        n55 = Unbundle By Name(w155) -> ("LB statusboolarray1.M123 Turbo Gate Valve closed"=w152:bool, "LB statusboolarray1.M123 Turbo Gate Valve opened"=w154:bool)
        n56 = Not(x=w154) -> (.not. x?=w153:bool)
        n57 = And(x=w152, y=w153) -> (x .and. y?=w151:bool)
        n58 = Concatenate Strings(w156, "-M123 Turbo Gate Valve is Open", "\n") -> (w149:string)
        n59 = Select(t="", s=w151, f=w149) -> (s? t:f=w159:string)
        n60 = Not(x=w151) -> (.not. x?=w148:bool)
      }
      frame "Is OAP Turbo Gate Valve Opened?" {
        n61 = Unbundle By Name(w167) -> ("LB statusboolarray1.OAP Turbo Gate Valve opened"=w164:bool, "LB statusboolarray1.OAP Turbo Gate Valve closed"=w166:bool)
        n62 = Not(x=w166) -> (.not. x?=w165:bool)
        n63 = And(x=w164, y=w165) -> (x .and. y?=w163:bool)
        n64 = Concatenate Strings(w168, "-OAP Turbo Gate Valve is NOT Open", "\n") -> (w160:string)
        n65 = Select(t="", s=w163, f=w160) -> (s? t:f=w171:string)
        n66 = Not(x=w163) -> (.not. x?=w162:bool)
      }
      frame "Is OAP Turbo Gate Valve Closed?" {
        n67 = Unbundle By Name(w179) -> ("LB statusboolarray1.OAP Turbo Gate Valve closed"=w176:bool, "LB statusboolarray1.OAP Turbo Gate Valve opened"=w178:bool)
        n68 = Not(x=w178) -> (.not. x?=w177:bool)
        n69 = And(x=w176, y=w177) -> (x .and. y?=w175:bool)
        n70 = Concatenate Strings(w180, "-OAP Turbo Gate Valve is Open", "\n") -> (w172:string)
        n71 = Select(t="", s=w175, f=w172) -> (s? t:f=w183:string)
        n72 = Not(x=w175) -> (.not. x?=w174:bool)
      }
      frame "Is BTLTurbo Gate Valve Opened?" {
        n73 = Unbundle By Name(w190) -> ("EC statusboolarray1.BTL Turbo Gate Valve opened"=w189:bool, "EC statusboolarray1.BTL Turbo Gate Valve closed"=w191:bool)
        n74 = Not(x=w191) -> (.not. x?=w188:bool)
        n75 = And(x=w189, y=w188) -> (x .and. y?=w187:bool)
        n76 = Concatenate Strings(w192, "-BTL Turbo Gate Valve is NOT Open", "\n") -> (w184:string)
        n77 = Select(t="", s=w187, f=w184) -> (s? t:f=w195:string)
        n78 = Not(x=w187) -> (.not. x?=w186:bool)
      }
      frame "Is BTL Turbo Gate Valve Closed?" {
        n79 = Unbundle By Name(w202) -> ("EC statusboolarray1.BTL Turbo Gate Valve closed"=w201:bool, "EC statusboolarray1.BTL Turbo Gate Valve opened"=w203:bool)
        n80 = Not(x=w203) -> (.not. x?=w200:bool)
        n81 = And(x=w201, y=w200) -> (x .and. y?=w199:bool)
        n82 = Concatenate Strings(w204, "-BTL Turbo Gate Valve is Open", "\n") -> (w196:string)
        n83 = Select(t="", s=w199, f=w196) -> (s? t:f=w207:string)
        n84 = Not(x=w199) -> (.not. x?=w198:bool)
      }
      frame "Is TARGET Turbo Gate Valve 1Opened?" {
        n85 = Unbundle By Name(w214) -> ("EC statusboolarray1.TARGET  Turbo Gate Valve 1 opened"=w213:bool, "EC statusboolarray1.TARGET  Turbo Gate Valve 1 closed"=w215:bool)
        n86 = Not(x=w215) -> (.not. x?=w212:bool)
        n87 = And(x=w213, y=w212) -> (x .and. y?=w211:bool)
        n88 = Concatenate Strings(w216, "-TARGET Turbo Gate Valve 1 is NOT Open", "\n") -> (w208:string)
        n89 = Select(t="", s=w211, f=w208) -> (s? t:f=w219:string)
        n90 = Not(x=w211) -> (.not. x?=w210:bool)
      }
      frame "Is TARGET1 Turbo Gate Valve Closed?" {
        n91 = Unbundle By Name(w226) -> ("EC statusboolarray1.TARGET  Turbo Gate Valve 1 closed"=w225:bool, "EC statusboolarray1.TARGET  Turbo Gate Valve 1 opened"=w227:bool)
        n92 = Not(x=w227) -> (.not. x?=w224:bool)
        n93 = And(x=w225, y=w224) -> (x .and. y?=w223:bool)
        n94 = Concatenate Strings(w228, "-TARGET Turbo Gate Valve 1 is Open", "\n") -> (w220:string)
        n95 = Select(t="", s=w223, f=w220) -> (s? t:f=w231:string)
        n96 = Not(x=w223) -> (.not. x?=w222:bool)
      }
      frame "Is TARGET Turbo Gate Valve 2 Opened?" {
        n97 = Unbundle By Name(w238) -> ("EC statusboolarray1.TARGET  Turbo Gate Valve 2 opened"=w237:bool, "EC statusboolarray1.TARGET  Turbo Gate Valve 2 closed"=w239:bool)
        n98 = Not(x=w239) -> (.not. x?=w236:bool)
        n99 = And(x=w237, y=w236) -> (x .and. y?=w235:bool)
        n100 = Concatenate Strings(w240, "-TARGET Turbo Gate Valve 2 is NOT Open", "\n") -> (w233:string)
        n101 = Select(t="", s=w235, f=w233) -> (s? t:f=w243:string)
        n102 = Not(x=w235) -> (.not. x?=w234:bool)
      }
      frame "Is TAREGT2 Turbo Gate Valve Closed?" {
        n103 = Unbundle By Name(w250) -> ("EC statusboolarray1.TARGET  Turbo Gate Valve 2 closed"=w249:bool, "EC statusboolarray1.TARGET  Turbo Gate Valve 2 opened"=w251:bool)
        n104 = Not(x=w251) -> (.not. x?=w248:bool)
        n105 = And(x=w249, y=w248) -> (x .and. y?=w247:bool)
        n106 = Concatenate Strings(w252, "-TARGET Turbo Gate Valve 2 is Open", "\n") -> (w245:string)
        n107 = Select(t="", s=w247, f=w245) -> (s? t:f=w255:string)
        n108 = Not(x=w247) -> (.not. x?=w246:bool)
      }
      frame "Is BTL2 Turbo Gate Valve Opened?" {
        n109 = Unbundle By Name(w262) -> ("EC statusboolarray1.BTL2 Turbo Gate Valve opened"=w261:bool, "EC statusboolarray1.BTL2 Turbo Gate Valve closed"=w263:bool)
        n110 = Not(x=w263) -> (.not. x?=w260:bool)
        n111 = And(x=w261, y=w260) -> (x .and. y?=w259:bool)
        n112 = Concatenate Strings(w264, "-BTL2 Turbo Gate Valve 2 is NOT Open", "\n") -> (w256:string)
        n113 = Select(t="", s=w259, f=w256) -> (s? t:f=w267:string)
        n114 = Not(x=w259) -> (.not. x?=w258:bool)
      }
      frame "Is BTL2 Turbo Gate Valve Closed?" {
        n115 = Unbundle By Name(w274) -> ("EC statusboolarray1.BTL2 Turbo Gate Valve closed"=w273:bool, "EC statusboolarray1.BTL2 Turbo Gate Valve opened"=w275:bool)
        n116 = Not(x=w275) -> (.not. x?=w272:bool)
        n117 = And(x=w273, y=w272) -> (x .and. y?=w271:bool)
        n118 = Concatenate Strings(w276, "-BTL2 Turbo Gate Valve 2 is Open", "\n") -> (w268:string)
        n119 = Select(t="", s=w271, f=w268) -> (s? t:f=w279:string)
        n120 = Not(x=w271) -> (.not. x?=w270:bool)
      }
      frame "Is HPD Turbo Gate Valve Opened?" {
        n121 = Unbundle By Name(w286) -> ("EC statusboolarray1.HPD  Turbo Gate Valve opened"=w285:bool, "EC statusboolarray1.HPD  Turbo Gate Valve closed"=w287:bool)
        n122 = Not(x=w287) -> (.not. x?=w284:bool)
        n123 = And(x=w285, y=w284) -> (x .and. y?=w283:bool)
        n124 = Concatenate Strings(w288, "-HPD Turbo Gate Valve 2 is NOT Open", "\n") -> (w280:string)
        n125 = Not(x=w283) -> (.not. x?=w282:bool)
        n126 = Select(t="", s=w283, f=w280) -> (s? t:f=w291:string)
      }
      frame "Is HPD Turbo Gate Valve Closed?" {
        n127 = Unbundle By Name(w298) -> ("EC statusboolarray1.HPD  Turbo Gate Valve closed"=w297:bool, "EC statusboolarray1.HPD  Turbo Gate Valve opened"=w299:bool)
        n128 = Not(x=w299) -> (.not. x?=w296:bool)
        n129 = And(x=w297, y=w296) -> (x .and. y?=w295:bool)
        n130 = Concatenate Strings(w300, "-HPD Turbo Gate Valve 2 is Open", "\n") -> (w292:string)
        n131 = Not(x=w295) -> (.not. x?=w294:bool)
        n132 = Select(t="", s=w295, f=w292) -> (s? t:f=w303:string)
      }
      frame "Is COMP to M123 gate Valve Opened?" {
        n133 = Unbundle By Name(w308) -> ("LB statusboolarray1.GATE VALVE COMP-M123 opened"=w310:bool, "LB statusboolarray1.GATE VALVE COMP-M123 closed"=w311:bool)
        n134 = Not(x=w311) -> (.not. x?=w309:bool)
        n135 = And(x=w310, y=w309) -> (x .and. y?=w307:bool)
        n136 = Concatenate Strings(w312, "-COMP to M123 Gate Valve is NOT Open", "\n") -> (w304:string)
        n137 = Select(t="", s=w307, f=w304) -> (s? t:f=w315:string)
        n138 = Not(x=w307) -> (.not. x?=w306:bool)
      }
      frame "Is COMP to M123 Valve Closed?" {
        n139 = Unbundle By Name(w320) -> ("LB statusboolarray1.GATE VALVE COMP-M123 closed"=w322:bool, "LB statusboolarray1.GATE VALVE COMP-M123 opened"=w323:bool)
        n140 = Not(x=w323) -> (.not. x?=w321:bool)
        n141 = And(x=w322, y=w321) -> (x .and. y?=w319:bool)
        n142 = Concatenate Strings(w324, "-COMP to M123 Gate Valve is Open", "\n") -> (w316:string)
        n143 = Select(t="", s=w319, f=w316) -> (s? t:f=w327:string)
        n144 = Not(x=w319) -> (.not. x?=w318:bool)
      }
      frame "Is HPBD Gate Valve Opened?" {
        n145 = Unbundle By Name(w332) -> ("LB statusboolarray1.GATE VALVE BEAM DUMP opened"=w334:bool, "LB statusboolarray1.GATE VALVE BEAM DUMP closed"=w335:bool)
        n146 = Not(x=w335) -> (.not. x?=w333:bool)
        n147 = And(x=w334, y=w333) -> (x .and. y?=w331:bool)
        n148 = Concatenate Strings(w336, "-BeamDump Gate Valve is NOT Open", "\n") -> (w329:string)
        n149 = Not(x=w331) -> (.not. x?=w328:bool)
        n150 = Select(t="", s=w331, f=w329) -> (s? t:f=w339:string)
      }
      frame "Is HPBD Gate Valve Closed?" {
        n151 = Unbundle By Name(w344) -> ("LB statusboolarray1.GATE VALVE BEAM DUMP closed"=w346:bool, "LB statusboolarray1.GATE VALVE BEAM DUMP opened"=w347:bool)
        n152 = Not(x=w347) -> (.not. x?=w345:bool)
        n153 = And(x=w346, y=w345) -> (x .and. y?=w343:bool)
        n154 = Concatenate Strings(w348, "-BeamDump Gate Valve is Open", "\n") -> (w341:string)
        n155 = Select(t="", s=w343, f=w341) -> (s? t:f=w351:string)
        n156 = Not(x=w343) -> (.not. x?=w340:bool)
      }
      frame "Is M123 to OAP gate valve opened?" {
        n157 = Unbundle By Name(w356) -> ("LB statusboolarray1.GATE VALVE M123-OAP opened"=w358:bool, "LB statusboolarray1.GATE VALVE M123-OAP closed"=w359:bool)
        n158 = Not(x=w359) -> (.not. x?=w357:bool)
        n159 = And(x=w358, y=w357) -> (x .and. y?=w355:bool)
        n160 = Concatenate Strings(w360, "-M123 to OAP Gate Valve is NOT Open", "\n") -> (w353:string)
        n161 = Select(t="", s=w355, f=w353) -> (s? t:f=w363:string)
        n162 = Not(x=w355) -> (.not. x?=w352:bool)
      }
      frame "Is M123 to OAP gate valve closed?" {
        n163 = Unbundle By Name(w368) -> ("LB statusboolarray1.GATE VALVE M123-OAP closed"=w370:bool, "LB statusboolarray1.GATE VALVE M123-OAP opened"=w371:bool)
        n164 = Not(x=w371) -> (.not. x?=w369:bool)
        n165 = And(x=w370, y=w369) -> (x .and. y?=w367:bool)
        n166 = Concatenate Strings(w372, "-M123 to OAP Gate Valve is NOT Open", "\n") -> (w365:string)
        n167 = Select(t="", s=w367, f=w365) -> (s? t:f=w375:string)
        n168 = Not(x=w367) -> (.not. x?=w364:bool)
      }
      frame "Is OAP to BLT gate valve opened?" {
        n169 = Unbundle By Name(w380) -> ("LB statusboolarray1.GATE VALVE OAP-BTL opened"=w382:bool, "LB statusboolarray1.GATE VALVE OAP-BTL closed"=w383:bool)
        n170 = Not(x=w383) -> (.not. x?=w381:bool)
        n171 = And(x=w382, y=w381) -> (x .and. y?=w377:bool)
        n172 = Concatenate Strings(w384, "-OAP to BLT Gate Valve is NOT Open", "\n") -> (w378:string)
        n173 = Select(t="", s=w377, f=w378) -> (s? t:f=w387:string)
        n174 = Not(x=w377) -> (.not. x?=w376:bool)
      }
      frame "Is OAP to BTL Gate Valve Closed?" {
        n175 = Unbundle By Name(w392) -> ("LB statusboolarray1.GATE VALVE OAP-BTL closed"=w394:bool, "LB statusboolarray1.GATE VALVE OAP-BTL opened"=w395:bool)
        n176 = Not(x=w395) -> (.not. x?=w393:bool)
        n177 = And(x=w394, y=w393) -> (x .and. y?=w389:bool)
        n178 = Concatenate Strings(w396, "-OAP to BLT Gate Valve is Open", "\n") -> (w390:string)
        n179 = Select(t="", s=w389, f=w390) -> (s? t:f=w399:string)
        n180 = Not(x=w389) -> (.not. x?=w388:bool)
      }
      frame "Is BLT to TARGET gate valve opened?" {
        n181 = Unbundle By Name(w404) -> ("EC statusboolarray1.GV BTL-TARGET opened"=w406:bool, "EC statusboolarray1.GV BTL-TARGET closed"=w407:bool)
        n182 = Not(x=w407) -> (.not. x?=w405:bool)
        n183 = And(x=w406, y=w405) -> (x .and. y?=w403:bool)
        n184 = Concatenate Strings(w408, "-BTL to TARGET Gate Valve is NOT Open", "\n") -> (w401:string)
        n185 = Select(t="", s=w403, f=w401) -> (s? t:f=w411:string)
        n186 = Not(x=w403) -> (.not. x?=w400:bool)
      }
      frame "Is BTL to TARGET Gate Valve Closed?" {
        n187 = Unbundle By Name(w416) -> ("EC statusboolarray1.GV BTL-TARGET closed"=w418:bool, "EC statusboolarray1.GV BTL-TARGET opened"=w419:bool)
        n188 = Not(x=w419) -> (.not. x?=w417:bool)
        n189 = And(x=w418, y=w417) -> (x .and. y?=w415:bool)
        n190 = Concatenate Strings(w420, "-BTL to TARGET Gate Valve is Open", "\n") -> (w413:string)
        n191 = Select(t="", s=w415, f=w413) -> (s? t:f=w423:string)
        n192 = Not(x=w415) -> (.not. x?=w412:bool)
      }
      frame "Is TARGET to BLT2 gate valve opened?" {
        n193 = Unbundle By Name(w428) -> ("EC statusboolarray1.GV TARGET-BTL2 opened"=w430:bool, "EC statusboolarray1.GV TARGET-BTL2 closed"=w431:bool)
        n194 = Not(x=w431) -> (.not. x?=w429:bool)
        n195 = And(x=w430, y=w429) -> (x .and. y?=w427:bool)
        n196 = Concatenate Strings(w432, "-TARGET to BLT2 Gate Valve is NOT Open", "\n") -> (w425:string)
        n197 = Select(t="", s=w427, f=w425) -> (s? t:f=w435:string)
        n198 = Not(x=w427) -> (.not. x?=w424:bool)
      }
      frame "Is TARGET to BTL2 Gate Valve Closed?" {
        n199 = Unbundle By Name(w440) -> ("EC statusboolarray1.GV TARGET-BTL2 closed"=w442:bool, "EC statusboolarray1.GV TARGET-BTL2 opened"=w443:bool)
        n200 = Not(x=w443) -> (.not. x?=w441:bool)
        n201 = And(x=w442, y=w441) -> (x .and. y?=w439:bool)
        n202 = Concatenate Strings(w444, "-TARGET to BLT2 Gate Valve is Open", "\n") -> (w437:string)
        n203 = Select(t="", s=w439, f=w437) -> (s? t:f=w447:string)
        n204 = Not(x=w439) -> (.not. x?=w436:bool)
      }
      frame "Is BLT2 to HPD gate valve opened?" {
        n205 = Unbundle By Name(w452) -> ("EC statusboolarray1.GV BTL2-HPD opened"=w454:bool, "EC statusboolarray1.GV BTL2-HPD closed"=w455:bool)
        n206 = Not(x=w455) -> (.not. x?=w453:bool)
        n207 = And(x=w454, y=w453) -> (x .and. y?=w451:bool)
        n208 = Concatenate Strings(w456, "-BLT2 to HPD Gate Valve is NOT Open", "\n") -> (w449:string)
        n209 = Select(t="", s=w451, f=w449) -> (s? t:f=w459:string)
        n210 = Not(x=w451) -> (.not. x?=w448:bool)
      }
      frame "Is BTL2 to HPD Gate Valve Closed?" {
        n211 = Unbundle By Name(w464) -> ("EC statusboolarray1.GV BTL2-HPD closed"=w466:bool, "EC statusboolarray1.GV BTL2-HPD opened"=w467:bool)
        n212 = Not(x=w467) -> (.not. x?=w465:bool)
        n213 = And(x=w466, y=w465) -> (x .and. y?=w463:bool)
        n214 = Concatenate Strings(w468, "-BLT2 to HPD Gate Valve is Open", "\n") -> (w461:string)
        n215 = Select(t="", s=w463, f=w461) -> (s? t:f=w471:string)
        n216 = Not(x=w463) -> (.not. x?=w460:bool)
      }
      frame "Is COMP at Atmospheric Pressure?" {
        n217 = Unbundle By Name(w477) -> ("LB statusintegerarray.COMP vacuum status word convectron ATM"=w474:i32)
        n218 = Equal To 0?(x=w474) -> (x = 0?=w473:bool)
        n219 = Concatenate Strings(w478, "-COMP is NOT at Atmospheric Pressure", "\n") -> (w475:string)
        n220 = Select(t="", s=w473, f=w475) -> (s? t:f=w481:string)
        n221 = Not(x=w473) -> (.not. x?=w472:bool)
      }
      frame "Is COMP at MID-VAC?" {
        n222 = Unbundle By Name(w488) -> ("LB statusintegerarray.COMP vacuum status word convectron ATM"=w485:i32)
        n223 = Equal?(x=w485, y=2) -> (x = y?=w483:bool)
        n224 = Concatenate Strings(w489, "-COMP is NOT at MID-VAC", "\n") -> (w486:string)
        n225 = Select(t="", s=w483, f=w486) -> (s? t:f=w492:string)
        n226 = Not(x=w483) -> (.not. x?=w482:bool)
      }
      frame "Is M123 at MID-VAC?" {
        n227 = Unbundle By Name(w499) -> ("LB statusintegerarray.M123 Convectron vacuum status word convectron"=w496:i32)
        n228 = Equal?(x=w496, y=2) -> (x = y?=w493:bool)
        n229 = Concatenate Strings(w500, "-M123 is NOT at MID-VAC", "\n") -> (w497:string)
        n230 = Select(t="", s=w493, f=w497) -> (s? t:f=w503:string)
        n231 = Not(x=w493) -> (.not. x?=w494:bool)
      }
      frame "Is M123 at Atmospheric Pressure?" {
        n232 = Unbundle By Name(w509) -> ("LB statusintegerarray.M123 vacuum status word convectron ATM"=w508:i32)
        n233 = Equal To 0?(x=w508) -> (x = 0?=w507:bool)
        n234 = Concatenate Strings(w510, "-M123 is NOT at Atmospheric Pressure", "\n") -> (w504:string)
        n235 = Select(t="", s=w507, f=w504) -> (s? t:f=w513:string)
        n236 = Not(x=w507) -> (.not. x?=w506:bool)
      }
      frame "Is BeamDump at Atmospheric Pressure?" {
        n237 = Unbundle By Name(w519) -> ("LB statusintegerarray.HPBD vacuum status word convectron ATM"=w518:i32)
        n238 = Equal To 0?(x=w518) -> (x = 0?=w515:bool)
        n239 = Concatenate Strings(w520, "-HPBD is NOT at Atmospheric Pressure", "\n") -> (w516:string)
        n240 = Select(t="", s=w515, f=w516) -> (s? t:f=w523:string)
        n241 = Not(x=w515) -> (.not. x?=w514:bool)
      }
      frame "Is OAP at Atmospheric Pressure?" {
        n242 = Unbundle By Name(w529) -> ("LB statusintegerarray.OAP vacuum status word convectron ATM"=w528:i32)
        n243 = Equal To 0?(x=w528) -> (x = 0?=w525:bool)
        n244 = Concatenate Strings(w530, "-OAP is NOT at Atmospheric Pressure", "\n") -> (w526:string)
        n245 = Select(t="", s=w525, f=w526) -> (s? t:f=w533:string)
        n246 = Not(x=w525) -> (.not. x?=w524:bool)
      }
      frame "Is OAP at MID-VAC?" {
        n247 = Unbundle By Name(w540) -> ("LB statusintegerarray.OAP vacuum status word convectron ATM"=w537:i32)
        n248 = Equal?(x=w537, y=2) -> (x = y?=w535:bool)
        n249 = Concatenate Strings(w541, "-OAP is NOT at MID-VAC", "\n") -> (w538:string)
        n250 = Select(t="", s=w535, f=w538) -> (s? t:f=w544:string)
        n251 = Not(x=w535) -> (.not. x?=w534:bool)
      }
      frame "Is BLT at Atmospheric Pressure" {
        n252 = Unbundle By Name(w547) -> ("EC statusintegerarray.BTL vacuum status word convectron ATM"=w550:i32)
        n253 = Equal To 0?(x=w550) -> (x = 0?=w546:bool)
        n254 = Concatenate Strings(w551, "-BTL is NOT at Atmospheric Pressure", "\n") -> (w548:string)
        n255 = Select(t="", s=w546, f=w548) -> (s? t:f=w554:string)
        n256 = Not(x=w546) -> (.not. x?=w545:bool)
      }
      frame "Is BTL at MID-VAC?" {
        n257 = Unbundle By Name(w559) -> ("EC statusintegerarray.BTL vacuum status word convectron ATM"=w558:i32)
        n258 = Equal?(x=w558, y=2) -> (x = y?=w556:bool)
        n259 = Concatenate Strings(w562, "-BTL is NOT at MID-VAC", "\n") -> (w560:string)
        n260 = Select(t="", s=w556, f=w560) -> (s? t:f=w565:string)
        n261 = Not(x=w556) -> (.not. x?=w555:bool)
      }
      frame "Is TARGET at Atmospheric Pressure?" {
        n262 = Unbundle By Name(w568) -> ("EC statusintegerarray.TARGET vacuum status word convectron ATM 2"=w571:i32)
        n263 = Equal To 0?(x=w571) -> (x = 0?=w567:bool)
        n264 = Concatenate Strings(w572, "-TARGET is NOT at Atmospheric Pressure", "\n") -> (w569:string)
        n265 = Select(t="", s=w567, f=w569) -> (s? t:f=w575:string)
        n266 = Not(x=w567) -> (.not. x?=w566:bool)
      }
      frame "Is TARGET at MID-VAC?" {
        n267 = Unbundle By Name(w580) -> ("EC statusintegerarray.TARGET vacuum status word convectron ATM 2"=w579:i32)
        n268 = Equal?(x=w579, y=2) -> (x = y?=w577:bool)
        n269 = Concatenate Strings(w583, "-TARGET is NOT at MID-VAC", "\n") -> (w581:string)
        n270 = Select(t="", s=w577, f=w581) -> (s? t:f=w586:string)
        n271 = Not(x=w577) -> (.not. x?=w576:bool)
      }
      frame "Is BLT2 at Atmospheric Pressure?" {
        n272 = Unbundle By Name(w589) -> ("EC statusintegerarray.BTL2 vacuum status word convectron ATM 3"=w592:i32)
        n273 = Equal To 0?(x=w592) -> (x = 0?=w588:bool)
        n274 = Concatenate Strings(w593, "-BTL2 is NOT at Atmospheric Pressure", "\n") -> (w590:string)
        n275 = Select(t="", s=w588, f=w590) -> (s? t:f=w596:string)
        n276 = Not(x=w588) -> (.not. x?=w587:bool)
      }
      frame "Is BTL2 at MID-VAC?" {
        n277 = Unbundle By Name(w601) -> ("EC statusintegerarray.BTL2 vacuum status word convectron ATM 3"=w600:i32)
        n278 = Concatenate Strings(w604, "-BTL2 is NOT at MID-VAC", "\n") -> (w602:string)
        n279 = Equal?(x=w600, y=2) -> (x = y?=w598:bool)
        n280 = Select(t="", s=w598, f=w602) -> (s? t:f=w607:string)
        n281 = Not(x=w598) -> (.not. x?=w597:bool)
      }
      frame "Is HPD at Atmospheric Pressure?" {
        n282 = Unbundle By Name(w610) -> ("EC statusintegerarray.HPD vacuum status word convectron ATM 4"=w613:i32)
        n283 = Equal To 0?(x=w613) -> (x = 0?=w609:bool)
        n284 = Concatenate Strings(w614, "-HPD is NOT at Atmospheric Pressure", "\n") -> (w611:string)
        n285 = Select(t="", s=w609, f=w611) -> (s? t:f=w617:string)
        n286 = Not(x=w609) -> (.not. x?=w608:bool)
      }
      frame "Is HPD at MID-VAC?" {
        n287 = Unbundle By Name(w622) -> ("EC statusintegerarray.HPD vacuum status word convectron ATM 4"=w621:i32)
        n288 = Equal?(x=w621, y=2) -> (x = y?=w619:bool)
        n289 = Concatenate Strings(w625, "-HPD is NOT at MID-VAC", "\n") -> (w623:string)
        n290 = Select(t="", s=w619, f=w623) -> (s? t:f=w628:string)
        n291 = Not(x=w619) -> (.not. x?=w618:bool)
      }
      frame "Is the EC Roughing Pump ON?" {
        n292 = Unbundle By Name(w633) -> ("EC statusboolarray2.ROUGHING PUMP run opened"=w629:bool)
        n293 = Concatenate Strings(w634, "-EC Roughing Pump is Not ON", "\n") -> (w632:string)
        n294 = Select(t="", s=w629, f=w632) -> (s? t:f=w637:string)
        n295 = Not(x=w629) -> (.not. x?=w630:bool)
      }
      frame "Is the EC Roughing Pump OFF?" {
        n296 = Unbundle By Name(w642) -> ("EC statusboolarray2.ROUGHING PUMP run opened"=w639:bool)
        n297 = Concatenate Strings(w643, "-EC Roughing Pump is NOT OFF", "\n") -> (w641:string)
        n298 = Select(t=w641, s=w639, f="") -> (s? t:f=w646:string)
        n299 = Not(x=w639) -> (.not. x?=w638:bool)
      }
      frame "Is the EC Backing Pump ON?" {
        n300 = Unbundle By Name(w651) -> ("EC statusboolarray2.BACKING PUMP run opened"=w647:bool)
        n301 = Concatenate Strings(w652, "-EC Backing Pump is NOT ON", "\n") -> (w648:string)
        n302 = Select(t="", s=w647, f=w648) -> (s? t:f=w655:string)
        n303 = Not(x=w647) -> (.not. x?=w650:bool)
      }
      frame "Is the EC Backing Pump OFF?" {
        n304 = Unbundle By Name(w660) -> ("EC statusboolarray2.BACKING PUMP run opened"=w659:bool)
        n305 = Concatenate Strings(w661, "-EC Backing Pump is NOT OFF", "\n") -> (w656:string)
        n306 = Select(t=w656, s=w659, f="") -> (s? t:f=w664:string)
        n307 = Not(x=w659) -> (.not. x?=w657:bool)
      }
      frame "Is the LB Roughing Pump ON?" {
        n308 = Unbundle By Name(w669) -> ("LB statusboolarray2.ROUGHING PUMP run"=w665:bool)
        n309 = Concatenate Strings(w670, "-LB Roughing Pump is Not ON", "\n") -> (w666:string)
        n310 = Select(t="", s=w665, f=w666) -> (s? t:f=w673:string)
        n311 = Not(x=w665) -> (.not. x?=w668:bool)
      }
      frame "Is the LB Roughing Pump Off?" {
        n312 = Unbundle By Name(w676) -> ("LB statusboolarray2.ROUGHING PUMP run"=w675:bool)
        n313 = Concatenate Strings(w679, "-LB Roughing Pump is ON", "\n") -> (w678:string)
        n314 = Select(t=w678, s=w675, f="") -> (s? t:f=w682:string)
        n315 = Not(x=w675) -> (.not. x?=w674:bool)
      }
      frame "Is the LB Backing Pump ON?" {
        n316 = Unbundle By Name(w687) -> ("LB statusboolarray2.BACKING PUMP run"=w686:bool)
        n317 = Concatenate Strings(w688, "-LB Backing Pump is NOT ON", "\n") -> (w683:string)
        n318 = Select(t="", s=w686, f=w683) -> (s? t:f=w691:string)
        n319 = Not(x=w686) -> (.not. x?=w685:bool)
      }
      frame "Is the LB Backing Pump OFF?" {
        n320 = Unbundle By Name(w696) -> ("LB statusboolarray2.BACKING PUMP run"=w693:bool)
        n321 = Concatenate Strings(w697, "-LB Backing Pump is NOT OFF", "\n") -> (w694:string)
        n322 = Select(t="", s=w693, f=w694) -> (s? t:f=w700:string)
        n323 = Not(x=w693) -> (.not. x?=w692:bool)
      }
      frame "Does the EC Roughing Pump have a fault?" {
        n324 = Unbundle By Name(w704) -> ("EC statusboolarray2.ROUGHING PUMP no fault closed"=w701:bool)
        n325 = Concatenate Strings(w705, "-EC Roughing Pump has a fault", "\n") -> (w702:string)
        n326 = Select(t=w702, s=w701, f="") -> (s? t:f=w708:string)
      }
      frame "Does the EC Backing Pump have a fault?" {
        n327 = Unbundle By Name(w712) -> ("EC statusboolarray2.BACKING PUMP no fault closed"=w709:bool)
        n328 = Concatenate Strings(w713, "-EC Backing Pump has a fault", "\n") -> (w710:string)
        n329 = Select(t=w710, s=w709, f="") -> (s? t:f=w716:string)
      }
      frame "Does the LB Roughing Pump have a fault?" {
        n330 = Unbundle By Name(w718) -> ("LB statusboolarray2.ROUGHING PUMP no fault"=w717:bool)
        n331 = Concatenate Strings(w721, "-LB Roughing Pump has a fault", "\n") -> (w719:string)
        n332 = Select(t=w719, s=w717, f="") -> (s? t:f=w724:string)
      }
      frame "Does the LB Backing Pump have a fault?" {
        n333 = Unbundle By Name(w726) -> ("LB statusboolarray2.BACKING PUMP no fault"=w725:bool)
        n334 = Concatenate Strings(w729, "-LB Backing Pump has a fault", "\n") -> (w727:string)
        n335 = Select(t=w727, s=w725, f="") -> (s? t:f=w732:string)
      }
      frame "Is the EC Backing Pipe at Atmospheric Pressure" {
        n336 = Unbundle By Name(w737) -> ("EC statusintegerarray.backing pump vacuum status word convectron"=w736:i32)
        n337 = Equal To 0?(x=w736) -> (x = 0?=w734:bool)
        n338 = Concatenate Strings(w738, "-EC Backing Pipe is NOT at Atmospheric Pressure", "\n") -> (w739:string)
        n339 = Select(t="", s=w734, f=w739) -> (s? t:f=w735:string)
        n340 = Not(x=w734) -> (.not. x?=w733:bool)
      }
      frame "Is the EC Backing Manifold at Atmospheric Pressure" {
        n341 = Unbundle By Name(w747) -> ("EC statusintegerarray.backing manifold vacuum status word convectron"=w746:i32)
        n342 = Equal To 0?(x=w746) -> (x = 0?=w744:bool)
        n343 = Concatenate Strings(w748, "-EC Backing Manifold is NOT at Atmospheric Pressure", "\n") -> (w749:string)
        n344 = Select(t="", s=w744, f=w749) -> (s? t:f=w745:string)
        n345 = Not(x=w744) -> (.not. x?=w743:bool)
      }
      frame "s the LB Backing Manifold at Atmospheric Pressure?" {
        n346 = Unbundle By Name(w755) -> ("LB statusintegerarray.backing manifold vacuum status word convectron"=w757:i32)
        n347 = Equal To 0?(x=w757) -> (x = 0?=w754:bool)
        n348 = Concatenate Strings(w758, "-LB Backing Manifold is NOT at Atmospheric Pressure", "\n") -> (w759:string)
        n349 = Select(t="", s=w754, f=w759) -> (s? t:f=w756:string)
        n350 = Not(x=w754) -> (.not. x?=w753:bool)
      }
      frame "Is the LB Backing Pipe at Atmospheric Pressure" {
        n351 = Unbundle By Name(w765) -> ("LB statusintegerarray.backing pump vacuum status word convectron"=w767:i32)
        n352 = Equal To 0?(x=w767) -> (x = 0?=w764:bool)
        n353 = Concatenate Strings(w768, "-LB Backing Pipe is NOT at Atmospheric Pressure", "\n") -> (w769:string)
        n354 = Select(t="", s=w764, f=w769) -> (s? t:f=w766:string)
        n355 = Not(x=w764) -> (.not. x?=w763:bool)
      }
      frame "Is the EC Roughing Pipe at Atmospheric Pressure" {
        n356 = Unbundle By Name(w778) -> ("EC statusintegerarray.roughing pump vacuum status word convectron"=w776:i32)
        n357 = Equal To 0?(x=w776) -> (x = 0?=w774:bool)
        n358 = Concatenate Strings(w777, "-EC Roughing Pipe is NOT at Atmospheric Pressure", "\n") -> (w779:string)
        n359 = Select(t="", s=w774, f=w779) -> (s? t:f=w775:string)
        n360 = Not(x=w774) -> (.not. x?=w773:bool)
      }
      frame "Is the EC Roughing Manifold at Atmospheric Pressure" {
        n361 = Unbundle By Name(w788) -> ("EC statusintegerarray.roughing manifold vacuum status word convectron"=w786:i32)
        n362 = Equal To 0?(x=w786) -> (x = 0?=w784:bool)
        n363 = Concatenate Strings(w787, "-EC Roughing Manifold is NOT at Atmospheric Pressure", "\n") -> (w789:string)
        n364 = Select(t="", s=w784, f=w789) -> (s? t:f=w785:string)
        n365 = Not(x=w784) -> (.not. x?=w783:bool)
      }
      frame "Is the LB Roughing Manifold at Atmospheric Pressure" {
        n366 = Unbundle By Name(w795) -> ("LB statusintegerarray.roughing manifold vacuum status word convectron"=w797:i32)
        n367 = Equal To 0?(x=w797) -> (x = 0?=w794:bool)
        n368 = Concatenate Strings(w798, "-LB Roughing Manifold is NOT at Atmospheric Pressure", "\n") -> (w799:string)
        n369 = Select(t="", s=w794, f=w799) -> (s? t:f=w796:string)
        n370 = Not(x=w794) -> (.not. x?=w793:bool)
      }
      frame "Is the LB Roughing Pipe at Atmospheric Pressure?" {
        n371 = Unbundle By Name(w808) -> ("EC statusintegerarray.roughing manifold vacuum status word convectron"=w806:i32)
        n372 = Equal To 0?(x=w806) -> (x = 0?=w804:bool)
        n373 = Concatenate Strings(w807, "-EC Roughing Manifold is NOT at Atmospheric Pressure", "\n") -> (w809:string)
        n374 = Not(x=w804) -> (.not. x?=w803:bool)
        n375 = Select(t="", s=w804, f=w809) -> (s? t:f=w805:string)
      }
      frame "Is LB Backing Manifold Valve Opened?" {
        n376 = Unbundle By Name(w819) -> ("LB statusboolarray1.BACKING MANIFOLD VALVE opened"=w821:bool, "LB statusboolarray1.BACKING MANIFOLD VALVE closed"=w822:bool)
        n377 = Not(x=w822) -> (.not. x?=w820:bool)
        n378 = And(x=w821, y=w820) -> (x .and. y?=w814:bool)
        n379 = Concatenate Strings(w818, "-LB Backing Manifold Valve is NOT Opened", "\n") -> (w816:string)
        n380 = Select(t="", s=w814, f=w816) -> (s? t:f=w817:string)
        n381 = Not(x=w814) -> (.not. x?=w813:bool)
      }
      frame "Is LB Roughing Manifold Valve Opened?" {
        n382 = Unbundle By Name(w831) -> ("LB statusboolarray1.ROUGHING MANIFOLD VALVE opened"=w833:bool, "LB statusboolarray1.ROUGHING MANIFOLD VALVE closed"=w834:bool)
        n383 = Not(x=w834) -> (.not. x?=w832:bool)
        n384 = And(x=w833, y=w832) -> (x .and. y?=w826:bool)
        n385 = Concatenate Strings(w830, "-LB Roughing Manifold Valve is NOT Opened", "\n") -> (w828:string)
        n386 = Select(t="", s=w826, f=w828) -> (s? t:f=w829:string)
        n387 = Not(x=w826) -> (.not. x?=w825:bool)
      }
      frame "Is EC Backing Manifold Valve Opened?" {
        n388 = Unbundle By Name(w841) -> ("EC statusboolarray1.BACKING MANIFOLD VALVE opened"=w845:bool, "EC statusboolarray1.BACKING MANIFOLD VALVE closed"=w846:bool)
        n389 = Not(x=w846) -> (.not. x?=w844:bool)
        n390 = And(x=w845, y=w844) -> (x .and. y?=w838:bool)
        n391 = Concatenate Strings(w843, "-EC Backing Manifold Valve is NOT Opened", "\n") -> (w839:string)
        n392 = Select(t="", s=w838, f=w839) -> (s? t:f=w842:string)
        n393 = Not(x=w838) -> (.not. x?=w837:bool)
      }
      frame "Is EC Roughing Manifold Valve Opened?" {
        n394 = Unbundle By Name(w853) -> ("EC statusboolarray1.ROUGHING MANIFOLD VALVE opened"=w857:bool, "EC statusboolarray1.ROUGHING MANIFOLD VALVE closed"=w858:bool)
        n395 = Not(x=w858) -> (.not. x?=w856:bool)
        n396 = And(x=w857, y=w856) -> (x .and. y?=w850:bool)
        n397 = Concatenate Strings(w855, "-EC Roughing Manifold Valve is NOT Opened", "\n") -> (w851:string)
        n398 = Select(t="", s=w850, f=w851) -> (s? t:f=w854:string)
        n399 = Not(x=w850) -> (.not. x?=w849:bool)
      }
      frame "Is COMP Roughing Valve Opened?" {
        n400 = Unbundle By Name(w863) -> ("LB statusboolarray1.COMPRESSOR ROUGHING VALVE opened"=w869:bool, "LB statusboolarray1.COMPRESSOR ROUGHING VALVE closed"=w870:bool)
        n401 = Not(x=w870) -> (.not. x?=w868:bool)
        n402 = And(x=w869, y=w868) -> (x .and. y?=w862:bool)
        n403 = Concatenate Strings(w867, "-COMP Roughing Valve is NOT Opened", "\n") -> (w864:string)
        n404 = Select(t="", s=w862, f=w864) -> (s? t:f=w866:string)
        n405 = Not(x=w862) -> (.not. x?=w861:bool)
      }
      frame "Is M123 Roughing Valve Opened?" {
        n406 = Unbundle By Name(w875) -> ("LB statusboolarray1.M123 ROUGHING VALVE opened"=w881:bool, "LB statusboolarray1.M123 ROUGHING VALVE closed"=w882:bool)
        n407 = Not(x=w882) -> (.not. x?=w880:bool)
        n408 = And(x=w881, y=w880) -> (x .and. y?=w874:bool)
        n409 = Concatenate Strings(w879, "-M123 Roughing Valve is NOT Opened", "\n") -> (w876:string)
        n410 = Select(t="", s=w874, f=w876) -> (s? t:f=w878:string)
        n411 = Not(x=w874) -> (.not. x?=w873:bool)
      }
      frame "Is M123 Roughing Valve Closed?" {
        n412 = Unbundle By Name(w890) -> ("LB statusboolarray1.M123 ROUGHING VALVE opened"=w888:bool, "LB statusboolarray1.M123 ROUGHING VALVE closed"=w886:bool)
        n413 = Not(x=w888) -> (.not. x?=w887:bool)
        n414 = And(x=w887, y=w886) -> (x .and. y?=w889:bool)
        n415 = Concatenate Strings(w894, "-M123 Roughing Valve is Not Closed", "\n") -> (w891:string)
        n416 = Select(t="", s=w889, f=w891) -> (s? t:f=w893:string)
        n417 = Not(x=w889) -> (.not. x?=w885:bool)
      }
      frame "Is OAP Roughing Valve Opened?" {
        n418 = Unbundle By Name(w899) -> ("LB statusboolarray1.OAP ROUGHING VALVE opened"=w905:bool, "LB statusboolarray1.OAP ROUGHING VALVE closed"=w906:bool)
        n419 = Not(x=w906) -> (.not. x?=w904:bool)
        n420 = And(x=w905, y=w904) -> (x .and. y?=w898:bool)
        n421 = Concatenate Strings(w903, "-OAP Roughing Valve is Closed", "\n") -> (w900:string)
        n422 = Select(t="", s=w898, f=w900) -> (s? t:f=w902:string)
        n423 = Not(x=w898) -> (.not. x?=w897:bool)
      }
      frame "Is OAP Roughing Valve Closed?" {
        n424 = Unbundle By Name(w911) -> ("LB statusboolarray1.OAP ROUGHING VALVE closed"=w917:bool, "LB statusboolarray1.OAP ROUGHING VALVE opened"=w918:bool)
        n425 = Not(x=w918) -> (.not. x?=w916:bool)
        n426 = And(x=w917, y=w916) -> (x .and. y?=w910:bool)
        n427 = Concatenate Strings(w915, "-OAP Roughing Valve is NOT Closed", "\n") -> (w912:string)
        n428 = Select(t="", s=w910, f=w912) -> (s? t:f=w914:string)
        n429 = Not(x=w910) -> (.not. x?=w909:bool)
      }
      frame "Is HPBD Roughing Valve Opened?" {
        n430 = Unbundle By Name(w923) -> ("LB statusboolarray1.BEAMDUMP ROUGHING VALVE opened"=w929:bool, "LB statusboolarray1.BEAMDUMP ROUGHING VALVE closed"=w930:bool)
        n431 = Not(x=w930) -> (.not. x?=w928:bool)
        n432 = And(x=w929, y=w928) -> (x .and. y?=w922:bool)
        n433 = Concatenate Strings(w927, "-BeamDump Roughing Valve is NOT Opened", "\n") -> (w924:string)
        n434 = Select(t="", s=w922, f=w924) -> (s? t:f=w926:string)
        n435 = Not(x=w922) -> (.not. x?=w921:bool)
      }
      frame "Is HPBD Roughing Valve Closed?" {
        n436 = Unbundle By Name(w935) -> ("LB statusboolarray1.BEAMDUMP ROUGHING VALVE closed"=w941:bool, "LB statusboolarray1.BEAMDUMP ROUGHING VALVE opened"=w942:bool)
        n437 = Not(x=w942) -> (.not. x?=w940:bool)
        n438 = And(x=w941, y=w940) -> (x .and. y?=w934:bool)
        n439 = Concatenate Strings(w939, "-BeamDump Roughing Valve is NOT Closed", "\n") -> (w936:string)
        n440 = Select(t="", s=w934, f=w936) -> (s? t:f=w938:string)
        n441 = Not(x=w934) -> (.not. x?=w933:bool)
      }
      frame "Is BTL Roughing Valve Opened?" {
        n442 = Unbundle By Name(w947) -> ("EC statusboolarray1.BTL ROUGHING VALVE opened"=w953:bool, "EC statusboolarray1.BTL ROUGHING VALVE closed"=w954:bool)
        n443 = Not(x=w954) -> (.not. x?=w952:bool)
        n444 = And(x=w953, y=w952) -> (x .and. y?=w946:bool)
        n445 = Concatenate Strings(w951, "-BTL Roughing Valve is Not Opened", "\n") -> (w948:string)
        n446 = Select(t="", s=w946, f=w948) -> (s? t:f=w950:string)
        n447 = Not(x=w946) -> (.not. x?=w945:bool)
      }
      frame "Is BTL Roughing Valve Closed?" {
        n448 = Unbundle By Name(w959) -> ("EC statusboolarray1.BTL ROUGHING VALVE closed"=w965:bool, "EC statusboolarray1.BTL ROUGHING VALVE opened"=w966:bool)
        n449 = Not(x=w966) -> (.not. x?=w964:bool)
        n450 = And(x=w965, y=w964) -> (x .and. y?=w958:bool)
        n451 = Concatenate Strings(w963, "-BTL Roughing Valve is NOT Closed", "\n") -> (w960:string)
        n452 = Select(t="", s=w958, f=w960) -> (s? t:f=w962:string)
        n453 = Not(x=w958) -> (.not. x?=w957:bool)
      }
      frame "Is TARGET Roughing Valve Opened?" {
        n454 = Unbundle By Name(w971) -> ("EC statusboolarray1.TARGET ROUGHING VALVE opened"=w977:bool, "EC statusboolarray1.TARGET ROUGHING VALVE closed"=w978:bool)
        n455 = Not(x=w978) -> (.not. x?=w976:bool)
        n456 = And(x=w977, y=w976) -> (x .and. y?=w970:bool)
        n457 = Concatenate Strings(w975, "-TARGET Roughing Valve is Not Opened", "\n") -> (w972:string)
        n458 = Select(t="", s=w970, f=w972) -> (s? t:f=w974:string)
        n459 = Not(x=w970) -> (.not. x?=w969:bool)
      }
      frame "Is TARGET Roughing Valve Closed?" {
        n460 = Unbundle By Name(w983) -> ("EC statusboolarray1.TARGET ROUGHING VALVE closed"=w989:bool, "EC statusboolarray1.TARGET ROUGHING VALVE opened"=w990:bool)
        n461 = Not(x=w990) -> (.not. x?=w988:bool)
        n462 = And(x=w989, y=w988) -> (x .and. y?=w982:bool)
        n463 = Concatenate Strings(w987, "-TARGET Roughing Valve is NOT Closed", "\n") -> (w984:string)
        n464 = Select(t="", s=w982, f=w984) -> (s? t:f=w986:string)
        n465 = Not(x=w982) -> (.not. x?=w981:bool)
      }
      frame "Is BTL2 Roughing Valve Opened?" {
        n466 = Unbundle By Name(w995) -> ("EC statusboolarray1.BTL2 ROUGHING VALVE opened"=w1001:bool, "EC statusboolarray1.BTL2 ROUGHING VALVE closed"=w1002:bool)
        n467 = Not(x=w1002) -> (.not. x?=w1000:bool)
        n468 = And(x=w1001, y=w1000) -> (x .and. y?=w994:bool)
        n469 = Concatenate Strings(w999, "-BTL2 Roughing Valve is NOT Opened", "\n") -> (w996:string)
        n470 = Not(x=w994) -> (.not. x?=w993:bool)
        n471 = Select(t="", s=w994, f=w996) -> (s? t:f=w998:string)
      }
      frame "Is BTL2 Roughing Valve Closed?" {
        n472 = Unbundle By Name(w1007) -> ("EC statusboolarray1.BTL2 ROUGHING VALVE closed"=w1013:bool, "EC statusboolarray1.BTL2 ROUGHING VALVE opened"=w1014:bool)
        n473 = Not(x=w1014) -> (.not. x?=w1012:bool)
        n474 = And(x=w1013, y=w1012) -> (x .and. y?=w1006:bool)
        n475 = Concatenate Strings(w1011, "-BTL2 Roughing Valve is NOT Closed", "\n") -> (w1008:string)
        n476 = Not(x=w1006) -> (.not. x?=w1005:bool)
        n477 = Select(t="", s=w1006, f=w1008) -> (s? t:f=w1010:string)
      }
      frame "Is HPD Roughing Valve Opened?" {
        n478 = Unbundle By Name(w1019) -> ("EC statusboolarray1.HPD ROUGHING VALVE opened"=w1025:bool, "EC statusboolarray1.HPD ROUGHING VALVE closed"=w1026:bool)
        n479 = Not(x=w1026) -> (.not. x?=w1024:bool)
        n480 = And(x=w1025, y=w1024) -> (x .and. y?=w1018:bool)
        n481 = Concatenate Strings(w1023, "-HPD Roughing Valve is NOT Opened", "\n") -> (w1020:string)
        n482 = Select(t="", s=w1018, f=w1020) -> (s? t:f=w1022:string)
        n483 = Not(x=w1018) -> (.not. x?=w1017:bool)
      }
      frame "Is HPD Roughing Valve Closed?" {
        n484 = Unbundle By Name(w1031) -> ("EC statusboolarray1.HPD ROUGHING VALVE closed"=w1037:bool, "EC statusboolarray1.HPD ROUGHING VALVE opened"=w1038:bool)
        n485 = Not(x=w1038) -> (.not. x?=w1036:bool)
        n486 = And(x=w1037, y=w1036) -> (x .and. y?=w1030:bool)
        n487 = Concatenate Strings(w1035, "-HPD Roughing Valve is NOT Closed", "\n") -> (w1032:string)
        n488 = Select(t="", s=w1030, f=w1032) -> (s? t:f=w1034:string)
        n489 = Not(x=w1030) -> (.not. x?=w1029:bool)
      }
      frame "Is COMP Turbo Backing Valve Opened?" {
        n490 = Unbundle By Name(w1043) -> ("LB statusboolarray1.COMPRESSOR Turbo Backing Valve opened"=w1049:bool, "LB statusboolarray1.COMPRESSOR Turbo Backing Valve closed"=w1050:bool)
        n491 = Not(x=w1050) -> (.not. x?=w1048:bool)
        n492 = And(x=w1049, y=w1048) -> (x .and. y?=w1041:bool)
        n493 = Concatenate Strings(w1047, "-COMP Turbo Backing Valve is Not Opened", "\n") -> (w1044:string)
        n494 = Select(t="", s=w1041, f=w1044) -> (s? t:f=w1046:string)
        n495 = Not(x=w1041) -> (.not. x?=w1042:bool)
      }
      frame "Is M123 Turbo Backing Valve Opened" {
        n496 = Unbundle By Name(w1055) -> ("LB statusboolarray1.M123 Turbo Backing Valve opened"=w1061:bool, "LB statusboolarray1.M123 Turbo Backing Valve closed"=w1062:bool)
        n497 = Not(x=w1062) -> (.not. x?=w1060:bool)
        n498 = And(x=w1061, y=w1060) -> (x .and. y?=w1053:bool)
        n499 = Concatenate Strings(w1059, "-M123 Turbo Backing Valve is Not Opened", "\n") -> (w1056:string)
        n500 = Select(t="", s=w1053, f=w1056) -> (s? t:f=w1058:string)
        n501 = Not(x=w1053) -> (.not. x?=w1054:bool)
      }
      frame "Is HPBD Turbo Backing Valve Opened?" {
        w1065 = FALSE ("BACKING PUMP no fault")
        n502 = Unbundle By Name(w1067) -> ("LB statusboolarray1.M123 Turbo Backing Valve opened"=w1073:bool, "LB statusboolarray1.M123 Turbo Backing Valve closed"=w1074:bool)
        n503 = Not(x=w1074) -> (.not. x?=w1072:bool)
        n504 = And(x=w1073, y=w1072) -> (x .and. y?=w1070:bool)
        n505 = Concatenate Strings(w1071, "-HPBD Turbo Backing Valve is Not Opened", "\n") -> (w1068:string)
        n506 = Select(t="", s=w1070, f=w1068) -> ()  [unwired: 1 out]
      }
      frame "Is OAP Turbo Backing Valve Opened?" {
        n507 = Unbundle By Name(w1080) -> ("LB statusboolarray1.OAP Turbo Backing Valve opened"=w1085:bool, "LB statusboolarray1.OAP Turbo Backing Valve closed"=w1086:bool)
        n508 = Not(x=w1086) -> (.not. x?=w1084:bool)
        n509 = And(x=w1085, y=w1084) -> (x .and. y?=w1077:bool)
        n510 = Concatenate Strings(w1083, "-OAP Turbo Backing Valve is NOT Opened", "\n") -> (w1081:string)
        n511 = Select(t="", s=w1077, f=w1081) -> (s? t:f=w1079:string)
        n512 = Not(x=w1077) -> (.not. x?=w1078:bool)
      }
      frame "Is BTL Turbo Backing Valve Opened?" {
        n513 = Unbundle By Name(w1092) -> ("EC statusboolarray1.BTL Turbo Backing Valve opened"=w1097:bool, "EC statusboolarray1.BTL Turbo Backing Valve closed"=w1098:bool)
        n514 = Not(x=w1098) -> (.not. x?=w1096:bool)
        n515 = And(x=w1097, y=w1096) -> (x .and. y?=w1089:bool)
        n516 = Concatenate Strings(w1095, "-BTL Turbo Backing Valve is NOT Opened", "\n") -> (w1093:string)
        n517 = Select(t="", s=w1089, f=w1093) -> (s? t:f=w1091:string)
        n518 = Not(x=w1089) -> (.not. x?=w1090:bool)
      }
      frame "Is TARGET1 Turbo Backing Valve Opened?" {
        n519 = Unbundle By Name(w1104) -> ("EC statusboolarray1.TARGET Turbo Backing Valve 1 opened"=w1109:bool, "EC statusboolarray1.TARGET Turbo Backing Valve 1 closed"=w1110:bool)
        n520 = Not(x=w1110) -> (.not. x?=w1108:bool)
        n521 = And(x=w1109, y=w1108) -> (x .and. y?=w1101:bool)
        n522 = Concatenate Strings(w1107, "-TARGET Turbo Backing Valve 1 is NOT Opened", "\n") -> (w1105:string)
        n523 = Select(t="", s=w1101, f=w1105) -> (s? t:f=w1103:string)
        n524 = Not(x=w1101) -> (.not. x?=w1102:bool)
      }
      frame "Is TARGET2 Turbo Backing Valve Opened?" {
        n525 = Unbundle By Name(w1116) -> ("EC statusboolarray1.TARGET Turbo Backing Valve 2 opened"=w1121:bool, "EC statusboolarray1.TARGET Turbo Backing Valve 2 closed"=w1122:bool)
        n526 = Not(x=w1122) -> (.not. x?=w1120:bool)
        n527 = And(x=w1121, y=w1120) -> (x .and. y?=w1113:bool)
        n528 = Concatenate Strings(w1119, "-TARGET Turbo Backing Valve 2 is NOT Opened", "\n") -> (w1117:string)
        n529 = Select(t="", s=w1113, f=w1117) -> (s? t:f=w1115:string)
        n530 = Not(x=w1113) -> (.not. x?=w1114:bool)
      }
      frame "Is BTL2 Turbo Backing Valve Opened?" {
        n531 = Unbundle By Name(w1128) -> ("EC statusboolarray1.BTL2 Turbo Backing Valve opened"=w1133:bool, "EC statusboolarray1.BTL2 Turbo Backing Valve closed"=w1134:bool)
        n532 = Not(x=w1134) -> (.not. x?=w1132:bool)
        n533 = And(x=w1133, y=w1132) -> (x .and. y?=w1125:bool)
        n534 = Concatenate Strings(w1131, "-BTL2 Turbo Backing Valve 2 is NOT Opened", "\n") -> (w1129:string)
        n535 = Select(t="", s=w1125, f=w1129) -> (s? t:f=w1127:string)
        n536 = Not(x=w1125) -> (.not. x?=w1126:bool)
      }
      frame "Is HPD Turbo Backing Valve Opened?" {
        n537 = Unbundle By Name(w1140) -> ("EC statusboolarray1.HPD Turbo Backing Valve opened"=w1145:bool, "EC statusboolarray1.HPD Turbo Backing Valve closed"=w1146:bool)
        n538 = Not(x=w1146) -> (.not. x?=w1144:bool)
        n539 = And(x=w1145, y=w1144) -> (x .and. y?=w1137:bool)
        n540 = Concatenate Strings(w1143, "-HPD Turbo Backing Valve 2 is NOT Opened", "\n") -> (w1141:string)
        n541 = Select(t="", s=w1137, f=w1141) -> (s? t:f=w1139:string)
        n542 = Not(x=w1137) -> (.not. x?=w1138:bool)
      }
      frame "Is M123 Backing at MID-VAC?" {
        n543 = Unbundle By Name(w1152) -> ("LB statusintegerarray.M123 Convectron vacuum status word convectron"=w1150:i32)
        n544 = Equal?(x=w1150, y=2) -> (x = y?=w1149:bool)
        n545 = Concatenate Strings(w1157, "-M123 Backing Pressure not at MID-VAC", "\n") -> (w1155:string)
        n546 = Select(t="", s=w1149, f=w1155) -> (s? t:f=w1154:string)
        n547 = Not(x=w1149) -> (.not. x?=w1153:bool)
      }
      frame "Is OAP Backing at MID-VAC?" {
        n548 = Unbundle By Name(w1163) -> ("LB statusintegerarray.OAP Convectron vacuum status word convectron"=w1161:i32)
        n549 = Equal?(x=w1161, y=2) -> (x = y?=w1160:bool)
        n550 = Concatenate Strings(w1168, "-OAP Backing Pressure not at MID-VAC", "\n") -> (w1166:string)
        n551 = Select(t="", s=w1160, f=w1166) -> (s? t:f=w1165:string)
        n552 = Not(x=w1160) -> (.not. x?=w1164:bool)
      }
      frame "Is TARGET1 Backing at MID-VAC?" {
        n553 = Unbundle By Name(w1172) -> ("EC statusintegerarray.TARGET1 Convectron vacuum status word convectron"=w1173:i32)
        n554 = Equal?(x=w1173, y=2) -> (x = y?=w1171:bool)
        n555 = Concatenate Strings(w1179, "-TARGET1 Backing Pressure not at MID-VAC", "\n") -> (w1177:string)
        n556 = Select(t="", s=w1171, f=w1177) -> (s? t:f=w1176:string)
        n557 = Not(x=w1171) -> (.not. x?=w1175:bool)
      }
      frame "Is TARGET2 Backing at MID-VAC?" {
        n558 = Unbundle By Name(w1183) -> ("EC statusintegerarray.TARGET2 Convectron vacuum status word convectron"=w1184:i32)
        n559 = Equal?(x=w1184, y=2) -> (x = y?=w1182:bool)
        n560 = Concatenate Strings(w1190, "-TARGET2 Backing Pressure not at MID-VAC", "\n") -> (w1188:string)
        n561 = Select(t="", s=w1182, f=w1188) -> (s? t:f=w1187:string)
        n562 = Not(x=w1182) -> (.not. x?=w1186:bool)
      }
      frame "Is BTL Backing at MID-VAC?" {
        n563 = Unbundle By Name(w1194) -> ("EC statusintegerarray.BTL Convectron vacuum status word convectron"=w1195:i32)
        n564 = Equal?(x=w1195, y=2) -> (x = y?=w1193:bool)
        n565 = Concatenate Strings(w1201, "-BTL Backing Pressure not at MID-VAC", "\n") -> (w1199:string)
        n566 = Select(t="", s=w1193, f=w1199) -> (s? t:f=w1198:string)
        n567 = Not(x=w1193) -> (.not. x?=w1197:bool)
      }
      frame "Is BTL2 Backing at MID-VAC?" {
        n568 = Unbundle By Name(w1205) -> ("EC statusintegerarray.BTL2 Convectron vacuum status word convectron"=w1206:i32)
        n569 = Equal?(x=w1206, y=2) -> (x = y?=w1204:bool)
        n570 = Concatenate Strings(w1212, "-BTL2 Backing Pressure not at MID-VAC", "\n") -> (w1210:string)
        n571 = Select(t="", s=w1204, f=w1210) -> (s? t:f=w1209:string)
        n572 = Not(x=w1204) -> (.not. x?=w1208:bool)
      }
      frame "Is HPD Backing at MID-VAC?" {
        n573 = Unbundle By Name(w1216) -> ("EC statusintegerarray.HPD Convectron vacuum status word convectron"=w1217:i32)
        n574 = Equal?(x=w1217, y=2) -> (x = y?=w1215:bool)
        n575 = Concatenate Strings(w1223, "-HPD Backing Pressure not at MID-VAC", "\n") -> (w1221:string)
        n576 = Select(t="", s=w1215, f=w1221) -> (s? t:f=w1220:string)
        n577 = Not(x=w1215) -> (.not. x?=w1219:bool)
      }
      frame "Is M123 Turbo in Normal Operation" {
        n578 = Unbundle By Name(w1227) -> ("LB statusintegerarray.M123 status word turbo pump"=w1228:i32)
        n579 = Equal?(x=w1228, y=2) -> (x = y?=w1226:bool)
        n580 = Concatenate Strings(w1234, "-M123 Turbo is NOT in Normal Running Mode", "\n") -> (w1232:string)
        n581 = Select(t="", s=w1226, f=w1232) -> (s? t:f=w1231:string)
        n582 = Not(x=w1226) -> (.not. x?=w1230:bool)
      }
      frame "Is COMP Turbo in Normal Operation" {
        n583 = Unbundle By Name(w1238) -> ("LB statusintegerarray.COMP status word turbo pump"=w1239:i32)
        n584 = Equal?(x=w1239, y=2) -> (x = y?=w1237:bool)
        n585 = Concatenate Strings(w1245, "-COMP Turbo is NOT in Normal Running Mode", "\n") -> (w1243:string)
        n586 = Select(t="", s=w1237, f=w1243) -> (s? t:f=w1242:string)
        n587 = Not(x=w1237) -> (.not. x?=w1241:bool)
      }
      frame "Is OAP Turbo in Normal Operation" {
        n588 = Unbundle By Name(w1249) -> ("LB statusintegerarray.OAP status word turbo pump"=w1250:i32)
        n589 = Equal?(x=w1250, y=2) -> (x = y?=w1248:bool)
        n590 = Concatenate Strings(w1256, "-OAP Turbo is NOT in Normal Running Mode", "\n") -> (w1254:string)
        n591 = Select(t="", s=w1248, f=w1254) -> (s? t:f=w1253:string)
        n592 = Not(x=w1248) -> (.not. x?=w1252:bool)
      }
      frame "Is BTL Turbo in Normal Operation" {
        n593 = Unbundle By Name(w1260) -> ("EC statusintegerarray.BTL status word turbo pump"=w1261:i32)
        n594 = Equal?(x=w1261, y=2) -> (x = y?=w1259:bool)
        n595 = Concatenate Strings(w1267, "-BTL Turbo is NOT in Normal Running Mode", "\n") -> (w1265:string)
        n596 = Select(t="", s=w1259, f=w1265) -> (s? t:f=w1264:string)
        n597 = Not(x=w1259) -> (.not. x?=w1263:bool)
      }
      frame "Is TARGET1 Turbo in Normal Operation" {
        n598 = Unbundle By Name(w1271) -> ("EC statusintegerarray.TARGET1 status word turbo pump"=w1272:i32)
        n599 = Equal?(x=w1272, y=2) -> (x = y?=w1270:bool)
        n600 = Concatenate Strings(w1278, "-TARGET1 Turbo is NOT in Normal Running Mode", "\n") -> (w1276:string)
        n601 = Select(t="", s=w1270, f=w1276) -> (s? t:f=w1275:string)
        n602 = Not(x=w1270) -> (.not. x?=w1274:bool)
      }
      frame "Is TARGET2 Turbo in Normal Operation" {
        n603 = Unbundle By Name(w1282) -> ("EC statusintegerarray.TARGET2 status word turbo pump"=w1283:i32)
        n604 = Equal?(x=w1283, y=2) -> (x = y?=w1281:bool)
        n605 = Concatenate Strings(w1289, "-TARGET2 Turbo is NOT in Normal Running Mode", "\n") -> (w1287:string)
        n606 = Select(t="", s=w1281, f=w1287) -> (s? t:f=w1286:string)
        n607 = Not(x=w1281) -> (.not. x?=w1285:bool)
      }
      frame "Is BTL2 Turbo in Normal Operation" {
        n608 = Unbundle By Name(w1293) -> ("EC statusintegerarray.BTL2 status word turbo pump??"=w1294:i32)
        n609 = Equal?(x=w1294, y=2) -> (x = y?=w1292:bool)
        n610 = Concatenate Strings(w1300, "-BTL2 Turbo is NOT in Normal Running Mode", "\n") -> (w1298:string)
        n611 = Select(t="", s=w1292, f=w1298) -> (s? t:f=w1297:string)
        n612 = Not(x=w1292) -> (.not. x?=w1296:bool)
      }
      frame "Is HPD Turbo in Normal Operation" {
        n613 = Unbundle By Name(w1304) -> ("EC statusintegerarray.HPD status word turbo pump"=w1305:i32)
        n614 = Equal?(x=w1305, y=2) -> (x = y?=w1303:bool)
        n615 = Concatenate Strings(w1311, "-HPD Turbo is NOT in Normal Running Mode", "\n") -> (w1309:string)
        n616 = Select(t="", s=w1303, f=w1309) -> (s? t:f=w1308:string)
        n617 = Not(x=w1303) -> (.not. x?=w1307:bool)
      }
    }
    n618 = Concatenate Strings(w32, w31) -> (w30:string)
  }
  "Msg out" <- w22
  "Results Array" <- w1
  "Convectron ATM Result Array" <- w4
  n619 = Empty Array?(array=w12) -> (empty?=w14:bool)
  n620 = Insert Into Array(array=w12, index=0, new element=w7) -> (w10:string[])
  n621 = And Array Elements(Boolean array=w6) -> (logical AND=→"Compound AND":bool)
  n622 = Or Array Elements(Boolean array=w6) -> (logical OR=→"Generate Event?":bool)
  n623 = Select(t=w12, s=w14, f=w10) -> (s? t:f=→"Status Array Out":string[])
